vi "WS1050 36 DUT Reliability HD_Cycling Ver1.4.vi"() -> ()   [LabVIEW 2012]
uses:
  WS_VCAP Driver 029/Source/WSVCAP Shell/Type Defs/WSVCAP SHL I2C DUT Mask Mode Enum.ctl
  <vilib>/Utility/file.llb/Read From Spreadsheet File (DBL).vi
  All Driver/Keithley/2012_Keithley 24XX/Keithley 24XX.lvlib
panel:
  out "VISA resource name out":refnum<visa-resource-name>="GPIB0::3::INSTR"
  out "error out 2":errorcluster={"status"=TRUE, "code"=-63192, "source"="niLvFpga_Open_PXI-7813R.vi"}
  in  "Reg1_Bit Cntrl":string[](array[string])=["01", "02", "04", "08", "10", "20", "40", "80", "03", "06", "0C", "D8", "33", "66", "CC", "07", "0E", "1C", "38", "70", "E0", "0F", "1E", "3C", "78", "F0", "1F", "3E", "7C", "F8", "3F", "7E", "FC", "7F", "FE", "FD", "FB", "F7", "EF", "DF", "BF", "7F", "FC", "F9", "F3", "E7", "CF", "9F", "3F", "F8", "F1", "E3", "C7", "8F", "1F", "F0", "E1", "C3", "87", "0F", "E0", "C1", "83", "07", "C0", "81", "03", "AA", "55", "00"]
  out "date string":string="5/19/2014"
  out "PS1 Out":refnum<visa-resource-name>
  out "Ke2000 Out":refnum<visa-resource-name>="GPIB0::9::INSTR"
  in  "VPI_Cmd":string[](array[string])=["000000", "3B3B3B", "000000"]
  in  "VPI Name":string[](array[string])=["All_Drivers OFF", "All Drivers ON", "All Drivers OFF2"]
  in  "Tab Control":T1(tab)
  in  "No of Cmd":i64=3
  in  "Board#":string="BRD5"
  in  "Serial Number":string[][](table)=[["DUT", "SN"], ["DUT1", "1"], ["DUT2", "2"], ["DUT3", "3"], ["DUT4", "4"], ["DUT5", "5"], ["DUT6", "6"], ["DUT7", "7"], ["DUT8", "8"], ["DUT9", "9"], ["DUT10", "10"], ["DUT11", "11"], ["DUT12", "12"], ["DUT13", "13"], ["DUT14", "14"], ["DUT15", "15"], ["DUT16", "16"], ["DUT17", "17"], ["DUT18", "18"], ["DUT19", "19"], ["DUT20", "20"], ["DUT21", "21"], ["DUT22", "22"], ["DUT23", "23"], ["DUT24", "24"], ["DUT25", "25"], ["DUT26", "26"], ["DUT27", "27"], ["DUT28", "28"], ["DUT29", "29"], ["DUT30", "30"], ["DUT31", "31"], ["DUT32", "32"], ["DUT33", "33"], ["DUT34", "34"], ["DUT35", "35"], ["DUT36", "36"]]
  in  "SPI Clock Rate (Hz)":dbl=5000000.0 caption="Cycle Speed" format="%.1p Hz"
  in  "Wafer#":string="T7-EB"
  in  "File Name":string="CYC_WS1050_T7_EB_65C_40V_25DC_EMPTY_BRD5_141017_1"
  in  "TMN DC\\CAP Data Log File Path":path=path "C:/WS1050 36 DUT Data"
  in  "Test Program":string="WS1050 36 DUT Reliability HD_Cycling Ver1.4"
  out "Current Date":string="8/28/2014"
  out "Current Time":string="0950"
  in  "Start Date":string="10/21/2014"
  in  "Start Time":string="1542"
  in  "Comment":string="CYC65C40V"
  in  "OK Button":bool
  in  "Calibration":bool
  in  "Verify CP":bool
  in  "CP Setting":i32(ring) items=["CP OFF", "CP ON", "CP 35V", "CP 40V", "DVA ON", "DVA OFF", "REG1 ON", "REG1 OFF", "REG2 ON", "REG2 OFF", "REG3 ON", "REG3 OFF"]
  in  "Stop Calibration":bool
  in  "Set VDD":dbl=3.3 format="%.3g"
  in  "Command":string[](array[string])=["07020100003B", "070201003B00", "0702013B0000"]
  in  "Clock Rate (Hz)":dbl=1000000.0 caption="Meas Speed" format="%.1p Hz"
  out "AR  Measurent(Hz)":dbl
  in  "PS1 Source":refnum<visa-resource-name>="GPIB0::5::INSTR"
  in  "Ke2000":refnum<visa-resource-name>="GPIB0::9::INSTR"
  in  "CP to HD/Cycle":i32(ring)=1 items=["CP HDC 35V", "CP HDC 40.25V", "CP HDC 27.5V", "CP HDC 30.5V", "CP HDC 44V"]
  out "Simulate FPGA":bool
  out "Online":bool
  out "AR Cycling(Hz)":dbl=5000000.0
  in  "Ke2400":refnum<visa-resource-name>="GPIB0::3::INSTR"
  in  "Initialize AD7747":bool
  in  "DUT Mask Mode":T2=enum."All"
  in  "RFFE Slave Address":u8=7 caption="Slave Address" format="0x%02x"
  out "Activity Log":string="05/19/2014 -- 12:24:35.853::WSVCAP::APP::Application Started\n05/19/2014 -- 12:24:37.606::WSVCAP::WSVCAP SHL::WR I2C-REG:0x0A;MASK:0xFFFFFFFFFFFF;C1 DATA:22:22:22:22:22:22:22:22:22:22:22:22:22:22:22:22;C2 DATA:22:22:22:22:22:22:22:22:22:22:22:22:22:22:22:22;C3 DATA:22:22:22:22:22:22:22:22:22:22:22:22:22:22:22:22\r\n05/19/2014 -- 12:24:37.773::WSVCAP::WSVCAP SHL::WR I2C-ST:0,0,4,1\r\n05/19/2014 -- 12:24:37.903::WSVCAP::WSVCAP SHL::RD I2C-BYTES:4;ADD:0x00;MASK:0xFFFFFFFFFFFF\r\n05/19/2014 -- 12:24:38.045::WSVCAP::WSVCAP SHL::RD I2C:C1 DATA:2:2:2:2:2:2:2:2:2:2:2:2:2:2:2:2|A7:A9:AA:82:82:7F:82:81:82:81:83:82:81:82:82:81|46:36:BB:88:44:A3:E9:2B:32:20:ED:25:BB:3D:68:B|2C:6A:EB:A7:22:56:FE:CC:36:82:D7:B0:3B:48:F9:CC;C2 DATA:2:2:2:2:2:2:2:2:2:2:2:2:2:2:2:2|94:94:94:80:80:80:80:80:81:7E:7E:81:80:7E:80:80|47:33:15:82:62:B:E8:1C:D7:C3:7D:41:7C:B7:4C:2A|C4:B4:AE:8:1E:D1:4E:37:11:C0:6F:63:42:9D:63:B5;C3 DATA:2:2:2:2:2:2:2:2:2:2:2:2:2:2:2:2|95:95:95:81:81:7E:81:80:84:7D:80:83:81:7E:7F:80|AB:C4:14:B5:7B:52:DF:C9:79:5D:5F:30:99:31:1E:F4|6E:5C:F7:A8:C3:EB:7B:EF:33:92:89:77:4D:67:75:DD;STATUS:0:0:4:0\r\n05/19/2014 -- 12:24:38.046::WSVCAP::WSVCAP SHL::WR I2C-REG:0x0A;MASK:0xFFFFFFFFFFFF;C1 DATA:22:22:22:22:22:22:22:22:22:22:22:22:22:22:22:22;C2 DATA:22:22:22:22:22:22:22:22:22:22:22:22:22:22:22:22;C3 DATA:22:22:22:22:22:22:22:22:22:22:22:22:22:22:22:22\r\n05/19/2014 -- 12:24:38.089::WSVCAP::WSVCAP SHL::WR I2C-ST:0,0,4,1\r\n05/19/2014 -- 12:24:38.219::WSVCAP::WSVCAP SHL::RD I2C-BYTES:4;ADD:0x00;MASK:0xFFFFFFFFFFFF\r\n05/19/2014 -- 12:24:38.362::WSVCAP::WSVCAP SHL::RD I2C:C1 DATA:2:2:2:2:2:2:2:2:2:2:2:2:2:2:2:2|A7:AB:AA:82:82:82:83:83:82:82:82:82:7F:82:82:81|4B:32:96:83:3E:61:43:17:25:62:AB:4D:A2:40:2E:5|3C:76:2B:B4:EE:E4:A9:1A:AA:A:26:C7:21:2E:87:5B;C2 DATA:2:2:2:2:2:2:2:2:2:2:2:2:2:2:2:2|94:94:94:80:80:80:80:80:80:7F:80:81:80:80:7F:80|4A:32:19:7D:19:6C:79:46:61:7F:4B:B8:A5:30:F3:14|B4:70:A:8C:9C:DC:43:FA:1E:A:C6:21:A:A9:13:F3;C3 DATA:2:2:2:2:2:2:2:2:2:2:2:2:2:2:2:2|95:97:94:81:80:81:82:81:80:7E:81:84:7F:81:80:80|B2:32:D0:A7:9E:4C:AB:D4:EE:D9:F0:82:B7:91:7:FF|C1:91:B6:3D:D8:E:1B:4F:9F:6A:F1:6C:E7:3F:7:BA;STATUS:0:0:4:0\r\n05/19/2014 -- 12:24:38.364::WSVCAP::WSVCAP SHL::WR I2C-REG:0x0A;MASK:0xFFFFFFFFFFFF;C1 DATA:22:22:22:22:22:22:22:22:22:22:22:22:22:22:22:22;C2 DATA:22:22:22:22:22:22:22:22:22:22:22:22:22:22:22:22;C3 DATA:22:22:22:22:22:22:22:22:22:22:22:22:22:22:22:22\r\n05/19/2014 -- 12:24:38.406::WSVCAP::WSVCAP SHL::WR I2C-ST:0,0,4,1\r\n05/19/2014 -- 12:24:38.536::WSVCAP::WSVCAP SHL::RD I2C-BYTES:4;ADD:0x00;MASK:0xFFFFFFFFFFFF\r\n05/19/2014 -- 12:24:38.678::WSVCAP::WSVCAP SHL::RD I2C:C1 DATA:2:2:2:2:2:2:2:2:2:2:2:2:2:2:2:2|A7:A9:AB:82:82:81:82:82:82:82:82:82:82:82:82:81|46:71:4C:87:43:3D:7F:FC:25:4F:8E:54:97:3E:60:8C|AA:F4:1F:B5:CE:43:1F:36:9:87:9C:78:86:5:B6:8E;C2 DATA:2:2:2:2:2:2:2:2:2:2:2:2:2:2:2:2|94:94:94:80:7F:7F:80:80:80:80:80:81:80:80:80:80|49:36:18:7D:6E:C5:E4:3C:81:2E:41:D3:75:71:E3:72|E8:D3:E6:D1:E0:48:AE:D4:54:D:E8:8E:B4:41:68:4;C3 DATA:2:2:2:2:2:2:2:2:2:2:2:2:2:2:2:2|95:95:95:81:7F:7F:81:81:81:81:81:84:81:81:82:81|B3:F5:90:AB:82:69:7B:93:D0:77:E8:D5:E8:8C:84:E8|B9:AC:EE:2B:B6:71:8F:4A:74:31:56:BB:8A:B7:A0:C8;STATUS:0:0:4:0\r\n05/19/2014 -- 12:24:38.681::WSVCAP::WSVCAP SHL::WR I2C-REG:0x0A;MASK:0xFFFFFFFFFFFF;C1 DATA:22:22:22:22:22:22:22:22:22:22:22:22:22:22:22:22;C2 DATA:22:22:22:22:22:22:22:22:22:22:22:22:22:22:22:22;C3 DATA:22:22:22:22:22:22:22:22:22:22:22:22:22:22:22:22\r\n05/19/2014 -- 12:24:38.723::WSVCAP::WSVCAP SHL::WR I2C-ST:0,0,4,1\r\n05/19/2014 -- 12:24:38.854::WSVCAP::WSVCAP SHL::RD I2C-BYTES:4;ADD:0x00;MASK:0xFFFFFFFFFFFF\r\n05/19/2014 -- 12:24:38.996::WSVCAP::WSVCAP SHL::RD I2C:C1 DATA:2:2:2:2:2:2:2:2:2:2:2:2:2:2:2:2|A7:A9:AA:82:82:7F:83:81:82:81:84:82:7F:82:7F:82|43:FB:E:7F:3C:AD:35:35:26:A2:6C:21:4B:3D:8:6|63:9A:E1:F3:95:32:91:42:90:3C:78:1F:5C:D7:5F:D8;C2 DATA:2:2:2:2:2:2:2:2:2:2:2:2:2:2:2:2|94:94:94:80:80:80:80:80:81:80:7E:81:80:7E:7F:80|48:36:18:7F:5E:3D:69:83:DE:AE:A1:9E:31:AE:BB:96|15:A0:44:17:13:FD:CC:C8:6D:B2:EF:A7:C:C7:3B:F;C3 DATA:2:2:2:2:2:2:2:2:2:2:2:2:2:2:2:2|95:96:94:81:81:7E:82:80:84:80:80:84:7F:7E:7D:82|AD:3B:6D:A9:7C:57:9D:F5:7A:96:23:5C:36:2D:ED:5A|CD:46:DB:3B:C7:BD:70:60:33:B8:B:F7:63:A:51:4D;STATUS:0:0:4:0\r\n05/19/2014 -- 12:24:38.998::WSVCAP::WSVCAP SHL::WR I2C-REG:0x0A;MASK:0xFFFFFFFFFFFF;C1 DATA:22:22:22:22:22:22:22:22:22:22:22:22:22:22:22:22;C2 DATA:22:22:22:22:22:22:22:22:22:22:22:22:22:22:22:22;C3 DATA:22:22:22:22:22:22:22:22:22:22:22:22:22:22:22:22\r\n05/19/2014 -- 12:24:39.040::WSVCAP::WSVCAP SHL::WR I2C-ST:0,0,4,1\r\n05/19/2014 -- 12:24:39.170::WSVCAP::WSVCAP SHL::RD I2C-BYTES:4;ADD:0x00;MASK:0xFFFFFFFFFFFF\r\n05/19/2014 -- 12:24:39.311::WSVCAP::WSVCAP SHL::RD I2C:C1 DATA:2:2:2:2:2:2:2:2:2:2:2:2:2:2:2:2|A7:AA:AB:82:82:81:82:81:82:81:82:82:82:82:7F:82|44:F1:90:87:45:44:C8:2C:2C:F1:FC:1B:94:3B:3C:75|4A:49:95:19:99:73:64:3:23:24:F3:A2:5E:7F:C4:B6;C2 DATA:2:2:2:2:2:2:2:2:2:2:2:2:2:2:2:2|94:94:94:80:80:80:80:7F:80:80:7E:80:80:7E:7F:80|4C:36:17:7D:A8:9F:DE:C7:53:6D:8A:F4:41:A5:C6:E0|90:2E:24:C:D9:22:E4:76:3B:40:1D:53:33:B1:3E:4D;C3 DATA:2:2:2:2:2:2:2:2:2:2:2:2:2:2:2:2|95:97:95:81:81:7F:81:80:80:81:7F:82:81:7E:7D:82|AE:2B:A7:AB:CC:CD:A4:38:FD:17:80:F2:92:2D:45:C4|76:E5:D:B9:AD:B5:BA:8D:28:32:9E:42:B7:20:4A:D9;STATUS:0:0:4:0\r\n05/19/2014 -- 12:24:39.313::WSVCAP::WSVCAP SHL::WR I2C-REG:0x0A;MASK:0xFFFFFFFFFFFF;C1 DATA:22:22:22:22:22:22:22:22:22:22:22:22:22:22:22:22;C2 DATA:22:22:22:22:22:22:22:22:22:22:22:22:22:22:22:22;C3 DATA:22:22:22:22:22:22:22:22:22:22:22:22:22:22:22:22\r\n05/19/2014 -- 12:24:39.355::WSVCAP::WSVCAP SHL::WR I2C-ST:0,0,4,1\r\n05/19/2014 -- 12:24:39.486::WSVCAP::WSVCAP SHL::RD I2C-BYTES:4;ADD:0x00;MASK:0xFFFFFFFFFFFF\r\n05/19/2014 -- 12:24:39.628::WSVCAP::WSVCAP SHL::RD I2C:C1 DATA:2:2:2:2:2:2:2:2:2:2:2:2:2:2:2:2|A7:A9:AA:82:82:82:83:82:82:82:82:82:7F:82:7F:82|47:18:E4:87:3E:E7:6:65:25:92:37:38:A8:3E:89:85|7C:A7:7:2B:A3:7A:EC:EF:89:ED:F4:D3:D8:BC:3A:F5;C2 DATA:2:2:2:2:2:2:2:2:2:2:2:2:2:2:2:2|94:94:94:80:7F:80:80:7F:81:80:7E:80:80:80:81:80|49:37:17:80:76:25:6A:F8:DF:55:97:4D:B8:5B:2B:B1|13:E3:9A:3E:1A:2D:4F:B6:DB:E9:61:FA:8B:D6:9:CC;C3 DATA:2:2:2:2:2:2:2:2:2:2:2:2:2:2:2:2|95:95:95:81:7F:80:82:81:84:80:7F:81:80:81:7F:82|AF:93:3B:AF:5B:11:82:E4:7E:C3:2D:72:9:96:D9:A|DB:96:F2:10:5F:64:9A:C6:98:12:27:7D:10:D3:20:D9;STATUS:0:0:4:0\r\n05/19/2014 -- 12:24:40.132::WSVCAP::WSVCAP SHL::CLOSE\r\n"
  in  "C1 Cap DAC":u8=128 caption="B Data In" format="0x%02x"
  in  "C2 Cap DAC":u8=128 caption="B Data In" format="0x%02x"
  in  "C3 Cap DAC":u8=128 caption="B Data In" format="0x%02x"
  out "IDD Brd(uA)":string
  in  "CP to Meas":i32(ring)=1 items=["CP HDC 35V", "CP HDC 40.25V", "CP HDC 27.5V", "CP HDC 30.5V", "CP HDC 44V"]
  in  "CP VPI":i32(ring) items=["CP HDC 35V", "CP HDC 40.25V", "CP HDC 27.5V", "CP HDC 30.5V", "CP HDC 44V"]
  in  "Repeat Meas(s)":u32=900
  in  "Real No. From\nLookup Table":bool
  in  "Control Panel":T3={"Verify Socket"=FALSE, "HD/CYC"=FALSE, "E-CAL"=FALSE, "DVA"=FALSE, "VPI"=TRUE, "VSA"=TRUE, "HS"=TRUE}
  out "Verify Socket":bool
  out "HD/CYC":bool
  out "E-CAL":bool
  out "DVA":bool
  out "VPI":bool
  out "VSA":bool
  out "HS":bool
  in  "Lot#":string="WS1050"
  out "AD7747 Values":string[][](table)
  in  "Freq(Hz)":string="12K"
  in  "Reset P/S":bool
  in  "WS1050/51":bool=TRUE
  in  "CP with DVA ON":i32(ring) items=["CP HDC 35V", "CP HDC 40.25V", "CP HDC 27.5V", "CP HDC 30.5V", "CP HDC 44V"]
  in  "% Duty Cycle":string="33"
  in  "Cmd To HD":string="0702013B3B3B"
  in  "Post CMd Delay":dbl[](array[numeric])=[1.8e-05, 1.8e-05, 1.8e-05] min=0.0 max=0.5 format="%#.0p s"
  in  "Cmin/Act":bool=TRUE
  in  "Test Seq":i32(ring)=3 items=["C1_C2_C3", "C2_C1_C3", "C3_C2_C1", "ALL"]
  out "40V_1":string[][](table)
  out "NOM IDD OFF(uA)":string
  out "40V_2":string[][](table)
  out "40V_3":string[][](table)
  out "Total Time":u64
  in  "Set HD/Cycle \nto Complete":u64=50000000000
  out "No of HD/Cycle\nCompleted":u64
  out "Cycle Count":u64 min=1 max=4 step=1
  out "Loop \ncompleted":i32=1
  out "Previous Time":string="12:20:26 PM"
  out "STATUS":string="Idle...."
  out "Total Delta C2(pF)":string[](array[string])
  out "Total Delta C1(pF)":string[](array[string])
  out "Total Delta C3(pF)":string[](array[string])
  out "RB Reg for HD":string[](array[string])
  out "RB Reg for HD/Cycle":string[](array[string])
  out "VPI C2":string[][](table)
  out "VPI C3":string[][](table)
  out "NOM IDD ON (uA)":string
  out "IDD_HD/CYC (uA)":string="164.601255E+0"
  in  "stop During HD/Cycles":bool
  in  "stop":bool
  out "IDD Stdby(uA)":string="2.606990E+0"
  out "VPI C1":string[][](table)
  out "VSA_V1":string[][](table)
  out "VSA_V2":string[][](table)
  out "VSA_V3":string[][](table)
  in  "VSA Voltage(V)":dbl[](array[numeric])=[-10.0, 0.0, 10.0]
  in  "DC_Temp":i32=65
  in  "HD/CYC Temp":i32=65
  in  "Time All ON (s)":u32=120
  in  "Time All OFF (s)":u32=120
  in  "HD_DC (Min)":u64=259200
  out "LPs Count":i32
  in  "X Repeat":i32=100
  out "No LPs to RP":i32
  out "Run Loops":i32=1
  out "TTCompleted":u64=2000
  in  "TTF Completed":u64=50000000000
  out "% Delta C_T0":string[][](array[string])
  out "% Delta C":string[][](array[string])
  out "EFuse RB T0":string[](array[string])
  out "Current EFuse Read back":string[](array[string])
  out "EFuse Readback Status":bool[](array[boolean])
  in  "DeltaC Target Setting(pF)":dbl=7.375
  out "error out":errorcluster
  in  "error in (no error)":errorcluster
  in  "HD RP":dbl=60.0
  in  "Cycle RP":dbl=10000.0
  out "Min Plot_1":dbl[][](graph) caption="(Y) Multi Plot 2"
  out "Min Plot_2":dbl[][](graph) caption="(Y) Multi Plot 2"
  out "Min Plot_3":dbl[][](graph) caption="(Y) Multi Plot 2"
  in  "Debug":bool
  in  "No of Rows\nFrom Spread Sheet":i32
  in  "Plot Delta Cmin":bool=TRUE
  in  "Plot":T4(ring)
  # "Company:  WiSpry Inc\n20 Fairbanks Ste 198 Irvine CA 92618\n\nAuthor:  Andy V Tran\nCreated:  04/21/2015\nLabVIEW 2012 Pro\nTest Program:  WS1050 36 DUT Reliability HD_Cycling ver1.4\nFPGA: WS_VCAP Driver 029"
  # "Note for HD Duty Cycle:\n1.  Set time to start HD_DC (Min), default is 259200 (6 months) \n2.  Set Time for Duty Cycle ON/OFF, default setting is 2 minutes\n3.  No of Loops to RP = 3600s/(Time ALL ON(s) + Time ALL + OFF(s))\n4.  Set X Repeat = no of runs, default is 100 runs\n5.  Set TTF Completed to stop the test.\n\nVer 1.4\n1.  Make measurement of C1, C2 and C3 at the same time"
  # "Minutes"
  # "X1000"
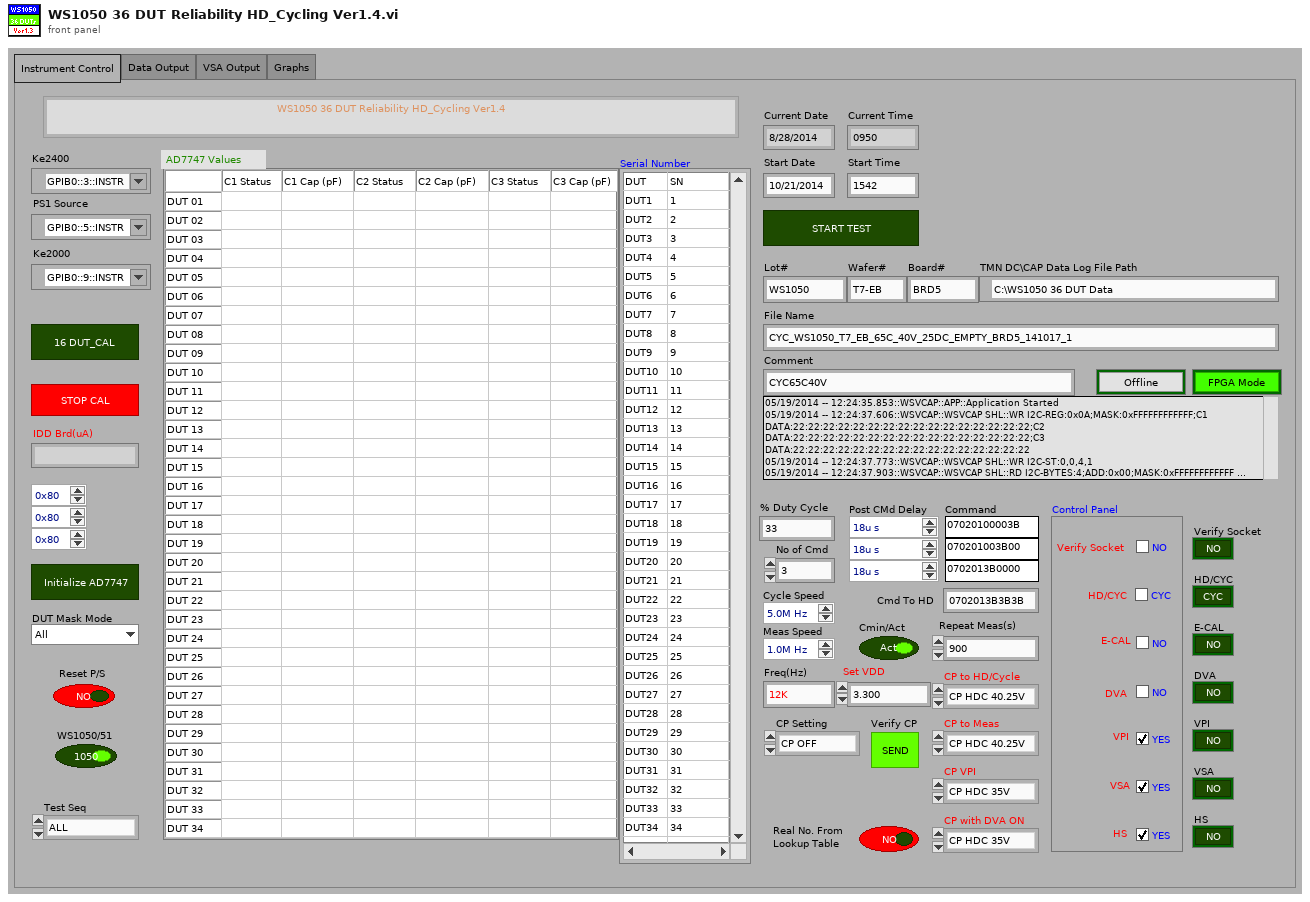
[diagram p1: front panel]
types:
  T1 = enum32{"Instrument Control", "Data Output", "VSA Output", "Graphs"}
  T2 = typedef "WSVCAP SHL I2C DUT Mask Mode Enum.ctl" = enum16{"Custom", "C1", "C2", "C3", "All"}
  T3 = cluster{"Verify Socket":bool, "HD/CYC":bool, "E-CAL":bool, "DVA":bool, "VPI":bool, "VSA":bool, "HS":bool}
  T4 = enum16{"ALL DUTs", "DUT 01", "DUT 02", "DUT 03", "DUT 04", "DUT 05", "DUT 06", "DUT 07", "DUT 08", "DUT 09", "DUT 10", "DUT 11", "DUT 12", "DUT 13", "DUT 14", "DUT 15", "DUT 16", "DUT 17", "DUT 18", "DUT 19", "DUT 20", "DUT 21", "DUT 22", "DUT 23", "DUT 24", "DUT 25", "DUT 26", "DUT 27", "DUT 28", "DUT 29", "DUT 30", "DUT 31", "DUT 32", "DUT 33", "DUT 34", "DUT 35", "DUT 36"}
  T5 = typedef "WSVCAP SHL Core System Cluster.ctl" = cluster{"Settings":T6, "FPGA Resource":tag, "Online":bool, "I2C Wait Ticks":u32, "SPI Wait Ticks":u32, "RFFE Wait Ticks":u32}
  T6 = typedef "WSVCAP SHL I2C Settings Cluster.ctl" = cluster{"FPGA Resource Name":string, "I2C Slave Address":u8, "I2C Clock Rate (Hz)":dbl, "SPI Clock Rate (Hz)":dbl, "RFFE Slave Address":u8, "RFFE Clock Rate (Hz)":dbl, "Simulate FPGA":bool, "C1 Cap DAC Default":u8, "C2 Cap DAC Default":u8, "C3 Cap DAC Default":u8}
  T7 = enum16{"Idle...", "Voltage 1", "Voltage 2", "Voltage 3"}[]
  T8 = cluster{"Test Program ":string, "Comment":string, "Data Out":string, "Data Out":string, "Data Out":string, string, "Data Out":string, "Data Out":string, "string":string, "Freq(Hz)":string, "Board#":string}
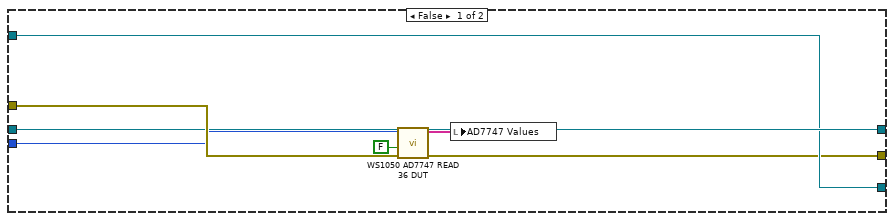
[diagram p10: hidden frame]
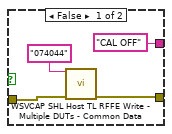
[diagram p11: hidden frame]
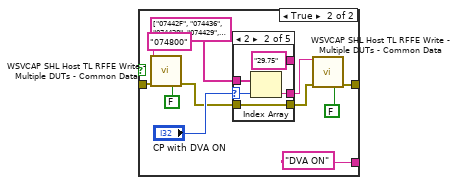
[diagram p12: hidden frame]
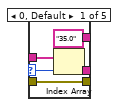
[diagram p13: hidden frame]
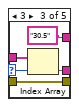
[diagram p14: hidden frame]
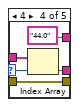
[diagram p15: hidden frame]
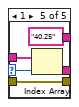
[diagram p16: hidden frame]
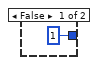
[diagram p17: hidden frame]
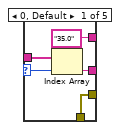
[diagram p18: hidden frame]
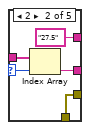
[diagram p19: hidden frame]
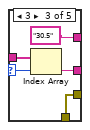
[diagram p20: hidden frame]
diagram:
  w19 = TRUE
  w25 = u16 0 items=["Off", "Moving Filter", "Repeating Filter"] ("Digital Filter (0: Off)")
  w26 = u16 7 items=["3.5 Digits"=4, "4.5 Digits"=5, "5.5 Digits"=6, "6.5 Digits"=7] ("Resolution (7: 6.5 digits)")
  n1 = case shown="True" w19 {
    tunnel: "error in (no error)" -> [w33 w34]
    tunnel: [w33 w41] -> w5
    frame False {
    }
    frame True {
      n2 = call "WSVCAP SHL Host TL Initialize.vi"("error in"=w34) -> ("error out"=w35:errorcluster)  [unwired: 13 in, 1 out]
      n3 = control-ref of="Activity Log"() -> (w37:refnum<vi>)
      n4 = call "ACT LG Activity Log Core.vi"("Display Ref"=w37, "Source"="WSVCAP", "Error In (no error)"=w35) -> ("Error Out"=w36:errorcluster)  [unwired: 11 in, 1 out]
      n5 = call "WSVCAP SHL Host TL Status Manager.vi"("error in"=w36) -> ("System Out"=w42:T5, "error out"=w41:errorcluster)  [unwired: 13 in]
      n6 = Unbundle By Name(w42) -> ("Online"=→"Online":bool, "Settings.Simulate FPGA"=→"Simulate FPGA":bool)
    }
  }
  n7 = case shown="True" TRUE {
    tunnel: w5 -> [w43 w48]
    tunnel: [w44 w47] -> w16
    tunnel: [w43 w46] -> w9
    tunnel: "Ke2400" -> [w44 w45]
    frame False {
    }
    frame True {
      n8 = VISA Write(VISA resource name=w45, write buffer="SOUR:FUNC VOLT;VOLT:MODE FIX;RANG 100;LEV 0.0;:SENS:FUNC \"CURR\";CURR:PROT 60E-3;RANG 100E-3;:OUTP ON", error in (no error)=w48) -> (VISA resource name out=w47:refnum<visa-resource-name>, error out=w46:errorcluster)  [unwired: 1 out]
    }
  }
  n9 = case shown="True" "Reset P/S" {
    tunnel: "PS1 Source" -> [w50 w57]
    tunnel: [w50 w55] -> w30
    tunnel: w5 -> [w51 w53]
    tunnel: [w51 w52] -> w4
    frame False {
    }
    frame True {
      n10 = call "Agilent 3631A Initialize.vi"("error in (no error)"=w53, "Default"=FALSE ("Reset? (T: Yes)"), "Reset"=TRUE ("ID Query? (T: Yes)"), "VISA resource name"=w57) -> ("error out"=w52:errorcluster, "VISA resource name out"=w55:refnum<visa-resource-name>)  [unwired: 6 in]
    }
  }
  n11 = call "Ke2000 Initialize.vi"("error in (no error)"=w5, "VISA resource name"="Ke2000") -> ("error out"=w27:errorcluster, "VISA resource name out"=w28:refnum<visa-resource-name>)  [unwired: 8 in]
  n12 = call "Ke2000 Configure DC Current.vi"("Resolution (7: 6.5 digits)"=w26, "Digital Filter (0: Off)"=w25, "Auto Range? (T: Auto)"=FALSE, "error in (no error)"=w27, "Custom Range (0 A)"=1.0, "VISA resource name"=w28) -> ("error out"=w6:errorcluster, "VISA resource name out"=w23:refnum<visa-resource-name>)  [unwired: 4 in]
  n13 = case shown="True" TRUE {
    tunnel: [_ w58] -> w32
    frame False {
    }
    frame True {
      n14 = call-poly <vilib>:"Read From Spreadsheet File.vi"("number of rows (all:-1)"=-1) -> ("all rows"=w58:dbl[][])  [unwired: 6 in, 4 out]
    }
  }
  n15 = Merge Errors(w9, w6, w4) -> (w17:errorcluster)
  n16 = while {
    tunnel: w17 -> [w62]
    tunnel: [w71] -> w13
    tunnel: w32 -> [w87]
    tunnel: w30 -> [w75]
    tunnel: w23 -> [w76]
    tunnel: [w85] -> w22
    tunnel: [w84] -> w21
    tunnel: w16 -> [w82]
    tunnel: [w81] -> w14
    tunnel: [FALSE ("stop")] -> w7
    i -> [w83]
    stop <- w88 stop-if-true
    n17 = case shown="0" w83 {
      tunnel: w62 -> [w99 w101]
      tunnel: [w98 w101] -> w78
      tunnel: "RFFE Slave Address" -> [w96 _]
      frame 0 {
        w92 = dbl[][] []
        w91 = "" ("uA")
        w93 = string[][] []
        w94 = string[] [] ("EFuse Read back")
        w100 = u64 0 ("No of HD/Cycle\nCompleted")
        n18 = local write "RB Reg for HD/Cycle"(w94) -> ()
        n19 = local write "Current EFuse Read back"(w94) -> ()
        n20 = local write "EFuse RB T0"(w94) -> ()
        n21 = local write "Total Delta C1(pF)"(w94) -> ()
        n22 = local write "Total Delta C2(pF)"(w94) -> ()
        n23 = local write "Total Delta C3(pF)"(w94) -> ()
        n24 = local write "No of HD/Cycle\nCompleted"(w100) -> ()
        n25 = local write "Cycle Count"(w100) -> ()
        n26 = local write "VPI C2"(w93) -> ()
        n27 = local write "VSA_V3"(w93) -> ()
        n28 = local write "VSA_V1"(w93) -> ()
        n29 = local write "40V_2"(w93) -> ()
        n30 = local write "40V_1"(w93) -> ()
        n31 = local write "NOM IDD OFF(uA)"(w91) -> ()
        n32 = local write "NOM IDD ON (uA)"(w91) -> ()
        n33 = local write "IDD Brd(uA)"(w91) -> ()
        n34 = local write "VSA_V2"(w93) -> ()
        n35 = local write "VPI C1"(w93) -> ()
        n36 = local write "VPI C3"(w93) -> ()
        n37 = local write "% Delta C"(w93) -> ()
        n38 = local write "% Delta C_T0"(w93) -> ()
        n39 = local write "40V_3"(w93) -> ()
        n40 = call "WSVCAP SHL Host TL RFFE Configure.vi"("RFFE Slave Address"=w96, "Clock Rate (Hz)"="Clock Rate (Hz)", "error in"=w99) -> ("Actual Rate (Hz)"=→"AR  Measurent(Hz)":dbl, "error out"=w98:errorcluster)  [unwired: 11 in]
        n41 = local write "Min Plot_3"(w92) -> ()
        n42 = local write "Min Plot_1"(w92) -> ()
        n43 = local write "Min Plot_2"(w92) -> ()
      }
      frame 1, Default {
      }
    }
    n44 = while {
      tunnel: ["stop"] -> w80
      tunnel: w78 -> [w127]
      tunnel: [w119] -> w72
      tunnel: w75 -> [w126]
      tunnel: w76 -> [w121]
      tunnel: [w122] -> w74
      tunnel: [w120] -> w73
      tunnel: [w117] -> w69
      tunnel: [w116] -> w68
      tunnel: [w115] -> w67
      tunnel: [w114] -> w66
      tunnel: [w113] -> w65
      tunnel: [w112] -> w64
      tunnel: [w111] -> w63
      tunnel: ["Command"] -> w61
      tunnel: ["Post CMd Delay"] -> w60
      stop <- w134 stop-if-true
      # "Set Date & Time to Start Test"
      n45 = case shown="True" "Initialize AD7747" {
        tunnel: w127 -> [w143 w148]
        tunnel: [w143 w144] -> w110
        tunnel: w126 -> [w142 w146]
        tunnel: [w142 w145] -> w125
        frame False {
        }
        frame True {
          w149 = T7 [enum."Voltage 2", enum."Voltage 3", enum."Voltage 1"] items=["Idle...", "Voltage 1", "Voltage 2", "Voltage 3"]
          n46 = for {
            tunnel: w146 -> [w159]
            tunnel: w149 -> [w157] mode=indexing
            tunnel: [w156] -> w145
            shift-right: [w152] -> w147
            shift-left: w148 -> [w160]
            n47 = local read "Set VDD"() -> (w155:dbl)
            n48 = call "E3631A_Voltage Controller.vi"("VISA resource name"=w159, "I_VDD(A)"=0.5, "Channel Controller"=w157, "Voltage 1"=w155, "Voltage 2"=3.3, "error in (no error)"=w160, "I_3.3V (A)"=0.5) -> ("VISA resource name out"=w156:refnum<visa-resource-name>, "error out"=w151:errorcluster)  [unwired: 7 in]
            n49 = call "Delay T4.vi"("milliseconds to wait"=u32 100, "error in (no error)"=w151) -> ("error out"=w152:errorcluster)  [unwired: 9 in]
          }
          n50 = call "WS1050_AD7747_Init 36DUT.vi"("error in"=w147) -> ("error out"=w144:errorcluster)  [unwired: 10 in]
        }
      }
      n51 = call "Time_stamp.vi"() -> ("date/time string"=w139:string, "date string"=w141:string)  [unwired: 2 in]
      "Current Date" <- w141
      "Current Time" <- w139
      n52 = Equal?(x=w141, y="Start Date") -> (x = y?=w137:bool)
      n53 = Equal?(x=w139, y="Start Time") -> (x = y?=w136:bool)
      n54 = And(x=w137, y=w136) -> (x .and. y?=w133:bool)
      n55 = Compound Arithmetic op=OR(w133, "OK Button", "stop") -> (w134:bool)
      n56 = case shown="True" "Calibration" {
        tunnel: w110 -> [w190 w207]
        tunnel: [w184 w204] -> w108
        tunnel: w125 -> [w189 w203]
        tunnel: "DUT Mask Mode" -> [w188 w199]
        tunnel: [w189 w198] -> w123
        tunnel: w121 -> [w187 w194]
        tunnel: [w187 w191] -> w120
        frame False {
          n57 = call "WS1050 AD7747 READ 36 DUT.vi"("error in"=w190, "Log (T)"=FALSE, "DUT Mask Mode (All)"=w188) -> ("error out"=w184:errorcluster, "AD7747 Values"=w185:string[][])  [unwired: 7 in]
          n58 = local write "AD7747 Values"(w185) -> ()
        }
        frame True {
          n59 = flat-sequence {
            tunnel: w207 -> [w216]
            tunnel: [w211] -> w206
            tunnel: w203 -> [w215]
            tunnel: [w214] -> w202
            tunnel: w199 -> [w213]
            tunnel: [w213] -> w200
            tunnel: w194 -> [w209]
            tunnel: [w208] -> w193
            tunnel: w206 -> [w240]
            tunnel: [w239] -> w205
            tunnel: w202 -> [w238]
            tunnel: [w238] -> w201
            tunnel: w200 -> [w237]
            tunnel: "C1 Cap DAC" -> [w233]
            tunnel: "C2 Cap DAC" -> [w232]
            tunnel: "C3 Cap DAC" -> [w231]
            tunnel: w193 -> [w230]
            tunnel: [w230] -> w192
            tunnel: w205 -> [w249]
            tunnel: [w252] -> w204
            tunnel: w201 -> [w251]
            tunnel: [w248] -> w198
            tunnel: w192 -> [w247]
            tunnel: [w247] -> w191
            frame #0 {
              w217 = T7 [enum."Voltage 2", enum."Voltage 3", enum."Voltage 1"] items=["Idle...", "Voltage 1", "Voltage 2", "Voltage 3"]
              n60 = for {
                tunnel: w215 -> [w228]
                tunnel: w217 -> [w226] mode=indexing
                tunnel: [w225] -> w214
                shift-right: [w223] -> w210
                shift-left: w216 -> [w229]
                n61 = local read "Set VDD"() -> (w220:dbl)
                n62 = call "E3631A_Voltage Controller.vi"("VISA resource name"=w228, "I_VDD(A)"=0.5, "Channel Controller"=w226, "Voltage 1"=w220, "Voltage 2"=3.3, "error in (no error)"=w229, "I_3.3V (A)"=0.5) -> ("VISA resource name out"=w225:refnum<visa-resource-name>, "error out"=w222:errorcluster)  [unwired: 7 in]
                n63 = call "Delay T4.vi"("milliseconds to wait"=u32 100, "error in (no error)"=w222) -> ("error out"=w223:errorcluster)  [unwired: 9 in]
              }
              n64 = call "Ke2000 Single Reading.vi"("error in (no error)"=w210, "VISA resource name"=w209) -> ("error out"=w211:errorcluster, "VISA resource name out"=w208:refnum<visa-resource-name>, "uA"=→"IDD Brd(uA)":string)  [unwired: 5 in, 2 out]
              n65 = One Button Dialog(message="Please verify all sockets should be empty...") -> ()  [unwired: 1 in, 1 out]
            }
            frame #1 {
              n66 = call "WS1050 CAPDAC Setting.vi"("DUT Mask Mode (All)"=w237, "error in"=w240, "C3 Cap DAC"=w231, "C2 Cap DAC"=w232, "C1 Cap DAC"=w233) -> ("error out"=w235:errorcluster)  [unwired: 5 in, 1 out]
              n67 = call "WS1050 OFFSET CAL.vi"("error in"=w235, "OFFSET CAL"=TRUE ("Read?")) -> ("error out"=w234:errorcluster)  [unwired: 8 in, 1 out]
              n68 = while {
                tunnel: w234 -> [w246]
                tunnel: [w245] -> w239
                tunnel: w237 -> [w243]
                stop <- "Stop Calibration" stop-if-true
                n69 = call "WS1050 AD7747 READ 36 DUT.vi"("error in"=w246, "Log (T)"=FALSE, "DUT Mask Mode (All)"=w243) -> ("error out"=w245:errorcluster, "AD7747 Values"=→"AD7747 Values":string[][])  [unwired: 7 in]
              }
            }
            frame #2 {
              w250 = T7 [enum."Voltage 2", enum."Voltage 3", enum."Voltage 1"] items=["Idle...", "Voltage 1", "Voltage 2", "Voltage 3"]
              n70 = for {
                tunnel: w251 -> [w264]
                tunnel: w250 -> [w261] mode=indexing
                tunnel: [w260] -> w248
                shift-right: [w256] -> w252
                shift-left: w249 -> [w262]
                n71 = call "E3631A_Voltage Controller.vi"("VISA resource name"=w264, "I_VDD(A)"=0.5, "Channel Controller"=w261, "Voltage 1"=0.0, "Voltage 2"=3.3, "error in (no error)"=w262, "I_3.3V (A)"=0.5) -> ("VISA resource name out"=w260:refnum<visa-resource-name>, "error out"=w255:errorcluster)  [unwired: 7 in]
                n72 = call "Delay T4.vi"("milliseconds to wait"=u32 100, "error in (no error)"=w255) -> ("error out"=w256:errorcluster)  [unwired: 9 in]
              }
              n73 = One Button Dialog(message="Calibration Completed....") -> ()  [unwired: 1 in, 1 out]
            }
          }
        }
      }
      n74 = call "Control Panel.vi"("error in (no error)"=w110, "Control Panel"="Control Panel") -> ("error out"=w107:errorcluster, "VPI"=w113:bool, "DVA"=w114:bool, "E-CAL"=w115:bool, "VSA"=w112:bool, "HD/CYC"=w116:bool, "HS"=w111:bool, "Verify Socket"=w117:bool)  [unwired: 2 in]
      "Verify Socket" <- w117
      "E-CAL" <- w115
      "VPI" <- w113
      "VSA" <- w112
      "HS" <- w111
      "HD/CYC" <- w116
      "DVA" <- w114
      n75 = Merge Errors(w107, w108) -> (w109:errorcluster)
      n76 = case shown="True" "Verify CP" {
        tunnel: [w161 w165] -> w119
        tunnel: w123 -> [w162 w168]
        tunnel: [w162 w166] -> w122
        tunnel: w109 -> [w161 w164]
        frame False {
        }
        frame True {
          w169 = T7 [enum."Voltage 2", enum."Voltage 3", enum."Voltage 1"] items=["Idle...", "Voltage 1", "Voltage 2", "Voltage 3"]
          # "Verify CP"
          n77 = for {
            tunnel: w168 -> [w182]
            tunnel: w169 -> [w180] mode=indexing
            shift-right: [w177] -> w167
            shift-left: w164 -> [w183]
            tunnel: [w175] -> w166
            n78 = local read "Set VDD"() -> (w179:dbl)
            n79 = call "E3631A_Voltage Controller.vi"("VISA resource name"=w182, "I_VDD(A)"=0.5, "Channel Controller"=w180, "Voltage 1"=w179, "Voltage 2"=3.3, "error in (no error)"=w183, "I_3.3V (A)"=0.5) -> ("VISA resource name out"=w175:refnum<visa-resource-name>, "error out"=w178:errorcluster)  [unwired: 7 in]
            n80 = call "Delay T4.vi"("milliseconds to wait"=u32 100, "error in (no error)"=w178) -> ("error out"=w177:errorcluster)  [unwired: 9 in]
          }
          n81 = Index Array(array=string[] ["074000", "074040", "07476F", "074776", "074800", "074820", "07413B", "074100", "07423B", "074200", "07433B", "074300"], index="CP Setting") -> (element=w170:string)
          n82 = call "WSVCAP SHL Host TL RFFE Write - Multiple DUTs - Common Data.vi"("Data Out"=w170, "error in"=w167, "Log (T)"=FALSE) -> ("error out"=w165:errorcluster)  [unwired: 12 in]
        }
      }
      n83 = Array Subset(array="Post CMd Delay", length="No of Cmd") -> (w105:dbl[])  [unwired: 1 in]
      n84 = Array Subset(array="Command", length="No of Cmd") -> (w106:string[])  [unwired: 1 in]
      n85 = property on="Post CMd Delay" class="Arr (strict)"("Number of Rows"="No of Cmd") -> ()  [unwired: 2 in, 2 out]
      n86 = local write "Command"(w106) -> ()
      n87 = local write "Post CMd Delay"(w105) -> ()
      n88 = property on="Command" class="Arr (strict)"("Number of Rows"="No of Cmd") -> ()  [unwired: 2 in, 2 out]
      n89 = Wait Until Next ms Multiple(millisecond multiple=u32 100) -> ()  [unwired: 1 out]
    }
    n90 = case shown="False" w80 {
      tunnel: w72 -> [w324 w1878]
      tunnel: [w309 w1878] -> w71
      tunnel: w87 -> [w325 _]
      tunnel: w74 -> [w323 w1876]
      tunnel: w73 -> [w315 w1877]
      tunnel: [w321 w1877] -> w85
      tunnel: [w319 w1876] -> w84
      tunnel: w82 -> [w312 w1875]
      tunnel: [w308 w1875] -> w81
      tunnel: "RFFE Slave Address" -> [w303 _]
      tunnel: [FALSE ("stop During HD/Cycles") FALSE ("stop During HD/Cycles")] -> w70
      tunnel: w69 -> [w278 _]
      tunnel: w68 -> [w277 _]
      tunnel: w67 -> [w276 _]
      tunnel: w66 -> [w275 _]
      tunnel: w65 -> [w274 _]
      tunnel: w64 -> [w273 _]
      tunnel: w63 -> [w272 _]
      tunnel: w61 -> [w266 _]
      tunnel: w60 -> [w265 _]
      frame False {
        w304 = u64 0 ("Total Completed")
        w283 = u32 100 ("milliseconds to wait")
        w320 = T7 [enum."Voltage 2", enum."Voltage 3", enum."Voltage 1"] items=["Idle...", "Voltage 1", "Voltage 2", "Voltage 3"]
        w322 = T7 [enum."Voltage 2", enum."Voltage 3", enum."Voltage 1"] items=["Idle...", "Voltage 1", "Voltage 2", "Voltage 3"]
        # "VSA"
        # "HS"
        # "HD/CYC"
        # "DVA"
        # "E-CAL"
        # "VPI"
        # "Verify Socket"
        n91 = for {
          tunnel: w324 -> [w1873]
          tunnel: w323 -> [w1872]
          tunnel: w322 -> [w1870] mode=indexing
          tunnel: [w1865] -> w317
          tunnel: [w1869] -> w307
          n92 = local read "Set VDD"() -> (w1868:dbl)
          n93 = call "E3631A_Voltage Controller.vi"("VISA resource name"=w1872, "I_VDD(A)"=0.5, "Channel Controller"=w1870, "Voltage 1"=w1868, "Voltage 2"=3.3, "error in (no error)"=w1873, "I_3.3V (A)"=0.5) -> ("VISA resource name out"=w1869:refnum<visa-resource-name>, "error out"=w1866:errorcluster)  [unwired: 7 in]
          n94 = call "Delay T4.vi"("milliseconds to wait"=u32 100, "error in (no error)"=w1866) -> ("error out"=w1865:errorcluster)  [unwired: 9 in]
        }
        n95 = local write "Total Time"(w304) -> ()
        n96 = local write "TTCompleted"(w304) -> ()
        n97 = call "WSVCAP SHL Host TL RFFE Write - Multiple DUTs - Common Data.vi"("Data Out"="074000", "error in"=w317, "Log (T)"=FALSE) -> ("error out"=w318:errorcluster)  [unwired: 12 in]
        n98 = local read "IDD Brd(uA)"() -> (w292:string)
        n99 = call "Delay T4.vi"("milliseconds to wait"=w283, "error in (no error)"=w318) -> ("error out"=w316:errorcluster)  [unwired: 9 in]
        n100 = call "Ke2000 Single Reading.vi"("error in (no error)"=w316, "VISA resource name"=w315) -> ("error out"=w293:errorcluster, "VISA resource name out"=w314:refnum<visa-resource-name>, "uA"=w295:string)  [unwired: 5 in, 2 out]
        n101 = call "Substration.vi"("error in (no error)"=w293, "Input2"=w292, "Input1"=w295) -> ("error out"=w268:errorcluster, "In1 - In2"=w294:string)  [unwired: 7 in]
        "IDD Stdby(uA)" <- w294
        n102 = case shown="True" w277 {
          tunnel: [1 ("X Repeat") w386] -> w306
          frame False {
          }
          frame True {
            n103 = local read "X Repeat"() -> (w386:i32)
          }
        }
        n104 = call "WSVCAP SHL Host TL RFFE Write - Multiple DUTs - Common Data.vi"("Data Out"="074040", "error in"=w268, "Log (T)"=FALSE) -> ("error out"=w267:errorcluster)  [unwired: 12 in]
        n105 = call "Delay T4.vi"("milliseconds to wait"=w283, "error in (no error)"=w267) -> ("error out"=w301:errorcluster)  [unwired: 9 in]
        n106 = case shown="False" w275 {
          tunnel: w301 -> [w348 w357]
          tunnel: [w347 w355] -> w299
          tunnel: ["DVA OFF" ("Data Out") "DVA ON" ("Data Out")] -> w300
          frame False {
            n107 = call "WSVCAP SHL Host TL RFFE Write - Multiple DUTs - Common Data.vi"("Data Out"="074820", "error in"=w348) -> ("error out"=w347:errorcluster)  [unwired: 13 in]
          }
          frame True {
            n108 = call "WSVCAP SHL Host TL RFFE Write - Multiple DUTs - Common Data.vi"("Data Out"="074800", "error in"=w357, "Log (T)"=FALSE) -> ("error out"=w353:errorcluster)  [unwired: 12 in]
            n109 = case shown="2" "CP with DVA ON" {
              selector: "CP with DVA ON" -> [w363 w368 w373 w378 w382]
              tunnel: string[] ["07442F", "074436", "074428", "074429", "07443B"] -> [w364 w369 w374 w379 w384]
              tunnel: [w362 w367 w372 w377 w383] -> w349
              tunnel: ["35.0" ("Data Out") "29.75" ("Data Out") "30.5" ("Data Out") "44.0" ("Data Out") "40.25" ("Data Out")] -> _
              tunnel: w353 -> [w360 w365 w370 w375 w380]
              tunnel: [w360 w365 w370 w375 w380] -> w352
              frame 0, Default {
                n110 = Index Array(array=w364, index=w363) -> (element=w362:string)
              }
              frame 2 {
                n111 = Index Array(array=w369, index=w368) -> (element=w367:string)
              }
              frame 3 {
                n112 = Index Array(array=w374, index=w373) -> (element=w372:string)
              }
              frame 4 {
                n113 = Index Array(array=w379, index=w378) -> (element=w377:string)
              }
              frame 1 {
                n114 = Index Array(array=w384, index=w382) -> (element=w383:string)
              }
            }
            n115 = call "WSVCAP SHL Host TL RFFE Write - Multiple DUTs - Common Data.vi"("Data Out"=w349, "error in"=w352, "Log (T)"=FALSE) -> ("error out"=w355:errorcluster)  [unwired: 12 in]
          }
        }
        n116 = for {
          N: 36 -> [_]
          tunnel: "Serial Number" -> [w330]
          tunnel: [w328] -> w280 mode=indexing
          i -> [w327]
          n117 = Increment(x=w327) -> (x+1=w326:i32)
          n118 = Index Array(array=w330, index (row)=w326, index (col)=1 ("disabled index (col)")) -> (element=w328:string)
        }
        n119 = Not(x=w272) -> (.not. x?=w279:bool)
        n120 = Number To Fractional String(number="Set VDD", precision (6)=i16 2) -> (F-format string=w297:string)  [unwired: 2 in]
        n121 = call "Delay T4.vi"("milliseconds to wait"=w283, "error in (no error)"=w299) -> ("error out"=w287:errorcluster)  [unwired: 9 in]
        n122 = case shown="True" w276 {
          tunnel: w287 -> [w334 w336]
          tunnel: [w331 w335] -> w286
          tunnel: ["CAL OFF" ("Data Out") "CAL ON" ("Data Out")] -> w288
          frame False {
            n123 = call "WSVCAP SHL Host TL RFFE Write - Multiple DUTs - Common Data.vi"("Data Out"="074044", "error in"=w334) -> ("error out"=w331:errorcluster)  [unwired: 13 in]
          }
          frame True {
            n124 = for {
              tunnel: string[] ["074900", "074920", "074900"] -> [w344] mode=indexing
              tunnel: w336 -> [w341]
              tunnel: [w340] -> w335
              n125 = call "WSVCAP SHL Host TL RFFE Write - Multiple DUTs - Common Data.vi"("Data Out"=w344, "error in"=w341, "Log (T)"=FALSE) -> ("error out"=w343:errorcluster)  [unwired: 12 in]
              n126 = call "Delay T4.vi"("milliseconds to wait"=u32 10, "error in (no error)"=w343) -> ("error out"=w340:errorcluster)  [unwired: 9 in]
            }
          }
        }
        n127 = for {
          N: w306 -> [_]
          tunnel: w325 -> [w424]
          tunnel: [w420] -> w321
          tunnel: w294 -> [w419]
          tunnel: w314 -> [w418]
          tunnel: "TMN DC\\CAP Data Log File Path" -> [w417]
          tunnel: w312 -> [w415]
          tunnel: [w414] -> w310
          tunnel: w307 -> [w389]
          shift-right: [w409] -> _
          shift-left: u64 0 -> [w411]
          tunnel: w277 -> [w408]
          tunnel: w303 -> [w403]
          tunnel: w303 -> [w402]
          tunnel: w300 -> [w401]
          tunnel: w297 -> [w400]
          tunnel: [w399] -> w291
          tunnel: w288 -> [w398]
          tunnel: w286 -> [w397]
          tunnel: w275 -> [w396]
          tunnel: w278 -> [w394]
          tunnel: w274 -> [w393]
          tunnel: w279 -> [w392]
          tunnel: w273 -> [w391]
          tunnel: w280 -> [w390]
          tunnel: [w389] -> w269
          tunnel: w266 -> [w388]
          tunnel: w265 -> [w387]
          i -> [w407]
          stop <- w395 stop-if-true
          n128 = while {
            tunnel: w424 -> [w650]
            tunnel: w417 -> [w661]
            tunnel: "Lot#" -> [w660]
            tunnel: "Wafer#" -> [w659]
            tunnel: w390 -> [w658]
            tunnel: "Test Program" -> [w657]
            tunnel: w390 -> [w656]
            tunnel: "Comment" -> [w655]
            tunnel: "Lot#" -> [w654]
            tunnel: "Wafer#" -> [w653]
            tunnel: w418 -> [w649]
            tunnel: [w652] -> w420
            tunnel: w419 -> [w648]
            tunnel: w415 -> [w645]
            tunnel: [w644] -> w414
            tunnel: [w552] -> w405
            tunnel: w407 -> [w590]
            tunnel: [w581] -> w409
            tunnel: w411 -> [w580]
            shift-right: [w579] -> _
            shift-left: u64 0 -> [w473]
            tunnel: [w578] -> w404
            tunnel: w408 -> [w576]
            tunnel: w403 -> [w551]
            tunnel: w402 -> [w549]
            tunnel: w401 -> [w497]
            tunnel: w400 -> [w495]
            tunnel: [w470] -> w399
            tunnel: w398 -> [w477]
            tunnel: w397 -> [w476]
            tunnel: w396 -> [w475]
            tunnel: w394 -> [w467]
            tunnel: w393 -> [w466]
            tunnel: w392 -> [w461]
            tunnel: w391 -> [w455]
            tunnel: w388 -> [w431]
            tunnel: w387 -> [w430]
            i -> [w577]
            stop <- w591 stop-if-true
            n129 = case shown="4" "CP to HD/Cycle" {
              selector: "CP to HD/Cycle" -> [w665 w670 w675 w680 w684]
              tunnel: string[] ["07476F", "074776", "074765", "074769", "07477B"] -> [w666 w671 w676 w681 w686]
              tunnel: [w664 w669 w674 w679 w685] -> w492
              tunnel: ["35.0" ("Data Out") "27.5" ("Data Out") "30.5" ("Data Out") "44.0" ("Data Out") "40.25" ("Data Out")] -> w491
              tunnel: [w662 w667 w672 w677 w682] -> w490
              tunnel: w476 -> [w662 w667 w672 w677 w682]
              frame 0, Default {
                n130 = Index Array(array=w666, index=w665) -> (element=w664:string)
              }
              frame 2 {
                n131 = Index Array(array=w671, index=w670) -> (element=w669:string)
              }
              frame 3 {
                n132 = Index Array(array=w676, index=w675) -> (element=w674:string)
              }
              frame 4 {
                n133 = Index Array(array=w681, index=w680) -> (element=w679:string)
              }
              frame 1 {
                n134 = Index Array(array=w686, index=w684) -> (element=w685:string)
              }
            }
            n135 = flat-sequence {
              tunnel: [w756] -> w643
              tunnel: [w751] -> w642
              tunnel: w650 -> [w754]
              tunnel: [w753] -> w641
              tunnel: w649 -> [w731]
              tunnel: w648 -> [w752]
              tunnel: [w752] -> w640
              tunnel: [w699] -> w639
              tunnel: [w696] -> w638
              tunnel: w490 -> [w744]
              tunnel: w590 -> [w749]
              tunnel: w577 -> [w723]
              tunnel: [w723] -> w587
              tunnel: w577 -> [w748]
              tunnel: w576 -> [w746]
              tunnel: [w745] -> w575
              tunnel: [w705] -> w570
              tunnel: [w704] -> w569
              tunnel: [w703] -> w568
              tunnel: [w709] -> w558
              tunnel: [w706] -> w557
              tunnel: w551 -> [w743]
              tunnel: [w743] -> w550
              tunnel: w549 -> [w742]
              tunnel: [w708] -> w536
              tunnel: [w707] -> w510
              tunnel: [w741] -> w498
              tunnel: w492 -> [w739]
              tunnel: [w725] -> w489
              tunnel: [w724] -> w481
              tunnel: w467 -> [w719]
              tunnel: w466 -> [w718]
              tunnel: [w718] -> w465
              tunnel: w461 -> [w717]
              tunnel: [w717] -> w460
              tunnel: w455 -> [w716]
              tunnel: [w716] -> w454
              tunnel: [w711] -> w449
              tunnel: ["Test Seq"] -> w445
              tunnel: "Real No. From\nLookup Table" -> [w702]
              tunnel: ["WS1050/51"] -> w439
              tunnel: ["Cmin/Act"] -> w435
              tunnel: w431 -> [w691]
              tunnel: w430 -> [w690]
              tunnel: [w689] -> w429
              tunnel: [w687] -> w425
              tunnel: w643 -> [w1076]
              tunnel: [w1072] -> w548
              tunnel: w642 -> [w1075]
              tunnel: w641 -> [w1081]
              tunnel: [w1081] -> w547
              tunnel: w640 -> [w1080]
              tunnel: w639 -> [w1074]
              tunnel: w638 -> [w1073]
              tunnel: [w1063] -> w546
              tunnel: [w1080] -> w545
              tunnel: [w1074] -> w544
              tunnel: [w1073] -> w543
              tunnel: w587 -> [w1078]
              tunnel: [w1078] -> w542
              tunnel: w575 -> [w1077]
              tunnel: [w1077] -> w541
              tunnel: [w1075] -> w540
              tunnel: w570 -> [w1071]
              tunnel: w569 -> [w1056]
              tunnel: w568 -> [w1057]
              tunnel: [w1068] -> w539
              tunnel: w558 -> [w1070]
              tunnel: w557 -> [w1068]
              tunnel: [w1064] -> w538
              tunnel: w550 -> [w1069]
              tunnel: [w1054] -> w537
              tunnel: w536 -> [w1054]
              tunnel: [w1056] -> w535
              tunnel: w510 -> [w1055]
              tunnel: [w1055] -> w509
              tunnel: [w1057] -> w507
              tunnel: w498 -> [w1067]
              tunnel: [w1066] -> w482
              tunnel: w481 -> [w1066]
              tunnel: w465 -> [w1062]
              tunnel: [w1062] -> w464
              tunnel: w460 -> [w1061]
              tunnel: [w1061] -> w459
              tunnel: w454 -> [w1060]
              tunnel: [w1060] -> w453
              tunnel: w449 -> [w1059]
              tunnel: [w1058] -> w448
              tunnel: w445 -> [w1052]
              tunnel: [w1052] -> w444
              tunnel: w439 -> [w1051]
              tunnel: [w1051] -> w438
              tunnel: w435 -> [w1050]
              tunnel: [w1050] -> w434
              tunnel: w429 -> [w1049]
              tunnel: [w1048] -> w428
              tunnel: [w1047] -> w427
              tunnel: w425 -> [w1045]
              tunnel: w548 -> [w1243]
              tunnel: [w1242] -> w534
              tunnel: w547 -> [w1254]
              tunnel: [w1254] -> w531
              tunnel: w546 -> [w1234]
              tunnel: [w1234] -> w529
              tunnel: w545 -> [w1253]
              tunnel: [w1253] -> w527
              tunnel: w544 -> [w1252]
              tunnel: [w1252] -> w525
              tunnel: w543 -> [w1251]
              tunnel: [w1251] -> w523
              tunnel: w542 -> [w1250]
              tunnel: [w1250] -> w521
              tunnel: w541 -> [w1249]
              tunnel: [w1249] -> w519
              tunnel: w540 -> [w1248]
              tunnel: [w1248] -> w517
              tunnel: w539 -> [w1247]
              tunnel: [w1247] -> w515
              tunnel: [w1239] -> w513
              tunnel: w538 -> [w1238]
              tunnel: w537 -> [w1245]
              tunnel: w535 -> [w1244]
              tunnel: w509 -> [w1231]
              tunnel: [w1231] -> w508
              tunnel: w507 -> [w1233]
              tunnel: [w1233] -> w506
              tunnel: [w1240] -> w505
              tunnel: [w1241] -> w483
              tunnel: w482 -> [w1241]
              tunnel: w464 -> [w1237]
              tunnel: [w1237] -> w463
              tunnel: w459 -> [w1236]
              tunnel: [w1236] -> w458
              tunnel: w453 -> [w1235]
              tunnel: [w1235] -> w452
              tunnel: w448 -> [w1232]
              tunnel: w444 -> [w1229]
              tunnel: [w1232] -> w443
              tunnel: [w1229] -> w442
              tunnel: w438 -> [w1228]
              tunnel: [w1228] -> w437
              tunnel: w434 -> [w1227]
              tunnel: [w1227] -> w433
              tunnel: w428 -> [w1226]
              tunnel: w427 -> [w1225]
              tunnel: [w1224] -> w426
              tunnel: w534 -> [w1342]
              tunnel: [w1341] -> w533
              tunnel: [w1337] -> w532
              tunnel: w531 -> [w1354]
              tunnel: [w1354] -> w530
              tunnel: w529 -> [w1331]
              tunnel: [w1331] -> w528
              tunnel: w527 -> [w1353]
              tunnel: [w1353] -> w526
              tunnel: w525 -> [w1352]
              tunnel: [w1352] -> w524
              tunnel: w523 -> [w1351]
              tunnel: [w1351] -> w522
              tunnel: w521 -> [w1350]
              tunnel: [w1350] -> w520
              tunnel: w519 -> [w1349]
              tunnel: [w1349] -> w518
              tunnel: w517 -> [w1348]
              tunnel: [w1348] -> w516
              tunnel: w515 -> [w1347]
              tunnel: [w1347] -> w514
              tunnel: w513 -> [w1346]
              tunnel: [w1346] -> w512
              tunnel: [w1328] -> w511
              tunnel: w508 -> [w1344]
              tunnel: w506 -> [w1343]
              tunnel: w505 -> [w1336]
              tunnel: ["DeltaC Target Setting(pF)"] -> w496
              tunnel: [w1339] -> w484
              tunnel: w483 -> [w1339]
              tunnel: w475 -> [w1338]
              tunnel: [w1338] -> w474
              tunnel: w463 -> [w1335]
              tunnel: [w1335] -> w462
              tunnel: w458 -> [w1334]
              tunnel: [w1334] -> w457
              tunnel: w452 -> [w1333]
              tunnel: [w1333] -> w451
              tunnel: w443 -> [w1332]
              tunnel: w442 -> [w1329]
              tunnel: [w1328] -> w440
              tunnel: w437 -> [w1327]
              tunnel: [w1327] -> w436
              tunnel: w433 -> [w1326]
              tunnel: [w1326] -> w432
              tunnel: w426 -> [w1325]
              tunnel: [w1473] -> w637
              tunnel: [w1440] -> w636
              tunnel: w533 -> [w1475]
              tunnel: w532 -> [w1454]
              tunnel: [w1463] -> w635
              tunnel: [w1454] -> w634
              tunnel: [w1424] -> w633
              tunnel: [w1422] -> w632
              tunnel: w530 -> [w1474]
              tunnel: [w1474] -> w631
              tunnel: w528 -> [w1463]
              tunnel: w526 -> [w1472]
              tunnel: [w1472] -> w630
              tunnel: w524 -> [w1468]
              tunnel: [w1468] -> w629
              tunnel: w522 -> [w1467]
              tunnel: [w1467] -> w628
              tunnel: w520 -> [w1464]
              tunnel: [w1464] -> w586
              tunnel: w518 -> [w1471]
              tunnel: [w1471] -> w574
              tunnel: w516 -> [w1470]
              tunnel: [w1469] -> w571
              tunnel: w514 -> [w1466]
              tunnel: w512 -> [w1462]
              tunnel: [w1423] -> w567
              tunnel: [w1465] -> w566
              tunnel: [w1462] -> w561
              tunnel: w511 -> [w1461]
              tunnel: [w1448] -> w556
              tunnel: [w1447] -> w555
              tunnel: [w1446] -> w554
              tunnel: w496 -> [w1460]
              tunnel: [w1445] -> w485
              tunnel: w484 -> [w1445]
              tunnel: [w1444] -> w480
              tunnel: w474 -> [w1443]
              tunnel: w462 -> [w1438]
              tunnel: w457 -> [w1437]
              tunnel: [w1437] -> w456
              tunnel: w451 -> [w1436]
              tunnel: [w1436] -> w450
              tunnel: w440 -> [w1433]
              tunnel: w436 -> [w1432]
              tunnel: w432 -> [w1427]
              tunnel: w637 -> [w1629]
              tunnel: [w1629] -> w627
              tunnel: [w1614] -> w626
              tunnel: [w1628] -> w625
              tunnel: w636 -> [w1627]
              tunnel: w635 -> [w1626]
              tunnel: w634 -> [w1625]
              tunnel: [w1626] -> w624
              tunnel: [w1625] -> w623
              tunnel: w633 -> [w1624]
              tunnel: [w1624] -> w622
              tunnel: w632 -> [w1623]
              tunnel: [w1623] -> w621
              tunnel: w631 -> [w1622]
              tunnel: [w1622] -> w620
              tunnel: w630 -> [w1621]
              tunnel: [w1621] -> w619
              tunnel: w629 -> [w1620]
              tunnel: [w1620] -> w618
              tunnel: w628 -> [w1619]
              tunnel: [w1619] -> w617
              tunnel: w645 -> [w1618]
              tunnel: [w1616] -> w616
              tunnel: [w1596] -> w615
              tunnel: [w1597] -> w614
              tunnel: [w1595] -> w613
              tunnel: w586 -> [w1612]
              tunnel: [w1612] -> w585
              tunnel: w574 -> [w1611]
              tunnel: [w1611] -> w573
              tunnel: w571 -> [w1628]
              tunnel: w567 -> [w1609]
              tunnel: w566 -> [w1610]
              tunnel: [w1610] -> w565
              tunnel: [w1609] -> w563
              tunnel: w561 -> [w1608]
              tunnel: [w1608] -> w560
              tunnel: w556 -> [w1594]
              tunnel: w555 -> [w1593]
              tunnel: w554 -> [w1592]
              tunnel: [w1589] -> w553
              tunnel: [w1594] -> w504
              tunnel: [w1593] -> w502
              tunnel: [w1592] -> w500
              tunnel: [w1591] -> w486
              tunnel: w485 -> [w1591]
              tunnel: w480 -> [w1590]
              tunnel: [w1590] -> w479
              tunnel: w456 -> [w1589]
              tunnel: w450 -> [w1588]
              tunnel: w627 -> [w1714]
              tunnel: [w1714] -> w612
              tunnel: w626 -> [w1738]
              tunnel: [w1737] -> w611
              tunnel: w661 -> [w1739]
              tunnel: w660 -> [w1736]
              tunnel: w659 -> [w1735]
              tunnel: w658 -> [w1734]
              tunnel: [w1733] -> w610
              tunnel: w625 -> [w1727]
              tunnel: [w1727] -> w609
              tunnel: w624 -> [w1732]
              tunnel: w623 -> [w1731]
              tunnel: [w1732] -> w608
              tunnel: [w1731] -> w607
              tunnel: [w1722] -> w606
              tunnel: w622 -> [w1730]
              tunnel: [w1730] -> w605
              tunnel: w621 -> [w1729]
              tunnel: [w1729] -> w604
              tunnel: w620 -> [w1726]
              tunnel: [w1728] -> w603
              tunnel: w473 -> [w1725]
              tunnel: [w1724] -> w602
              tunnel: [w1712] -> w601
              tunnel: w619 -> [w1723]
              tunnel: w618 -> [w1721]
              tunnel: w617 -> [w1720]
              tunnel: "File Name" -> [w1719]
              tunnel: w616 -> [w1718]
              tunnel: [w1718] -> w600
              tunnel: w615 -> [w1717]
              tunnel: [w1717] -> w599
              tunnel: [w1716] -> w598
              tunnel: w614 -> [w1716]
              tunnel: w613 -> [w1715]
              tunnel: [w1715] -> w597
              tunnel: [w1710] -> w588
              tunnel: w585 -> [w1711]
              tunnel: [w1711] -> w583
              tunnel: w580 -> [w1709]
              tunnel: w573 -> [w1708]
              tunnel: [w1708] -> w572
              tunnel: w565 -> [w1707]
              tunnel: [w1707] -> w564
              tunnel: w563 -> [w1706]
              tunnel: [w1706] -> w562
              tunnel: w560 -> [w1705]
              tunnel: [w1705] -> w559
              tunnel: w553 -> [w1704]
              tunnel: w504 -> [w1703]
              tunnel: [w1703] -> w503
              tunnel: w502 -> [w1702]
              tunnel: [w1702] -> w501
              tunnel: w500 -> [w1701]
              tunnel: [w1701] -> w499
              tunnel: w489 -> [w1700]
              tunnel: [w1700] -> w488
              tunnel: [w1699] -> w487
              tunnel: w486 -> [w1699]
              tunnel: w479 -> [w1698]
              tunnel: [w1698] -> w478
              tunnel: ["Freq(Hz)"] -> w447
              tunnel: ["Board#"] -> w446
              tunnel: w612 -> [w1811]
              tunnel: w611 -> [w1810]
              tunnel: w661 -> [w1773]
              tunnel: w657 -> [w1805]
              tunnel: w656 -> [w1808]
              tunnel: w655 -> [w1804]
              tunnel: w654 -> [w1807]
              tunnel: w653 -> [w1803]
              tunnel: w610 -> [w1806]
              tunnel: [w1811] -> w593
              tunnel: [w1809] -> w594
              tunnel: w609 -> [w1801]
              tunnel: [w1801] -> w595
              tunnel: w608 -> [w1800]
              tunnel: w607 -> [w1785]
              tunnel: w606 -> [w1799]
              tunnel: w605 -> [w1798]
              tunnel: w604 -> [w1787]
              tunnel: [w1795] -> w596
              tunnel: w603 -> [w1797]
              tunnel: w602 -> [w1796]
              tunnel: w601 -> [w1795]
              tunnel: "File Name" -> [w1766]
              tunnel: w600 -> [w1794]
              tunnel: [w1794] -> w592
              tunnel: w599 -> [w1793]
              tunnel: w598 -> [w1792]
              tunnel: w597 -> [w1791]
              tunnel: [w1790] -> w589
              tunnel: w588 -> [w1790]
              tunnel: [w1769] -> w584
              tunnel: w583 -> [w1769]
              tunnel: w572 -> [w1789]
              tunnel: w564 -> [w1788]
              tunnel: w562 -> [w1786]
              tunnel: w559 -> [w1784]
              tunnel: w503 -> [w1783]
              tunnel: w501 -> [w1782]
              tunnel: w499 -> [w1781]
              tunnel: w497 -> [w1780]
              tunnel: w477 -> [w1779]
              tunnel: w491 -> [w1778]
              tunnel: w495 -> [w1777]
              tunnel: w488 -> [w1776]
              tunnel: w487 -> [w1775]
              tunnel: w478 -> [w1774]
              tunnel: [w1771] -> w472
              tunnel: [w1762] -> w468
              tunnel: w447 -> [w1761]
              tunnel: w446 -> [w1759]
              tunnel: [w1832] -> w651
              tunnel: [w1833] -> w652
              tunnel: [w1834] -> w552
              tunnel: w596 -> [w1825]
              tunnel: w595 -> [w1833]
              tunnel: w594 -> [w1820]
              tunnel: w593 -> [w1834]
              tunnel: w592 -> [w1827]
              tunnel: [w1827] -> w644
              tunnel: [w1824] -> w581
              tunnel: w589 -> [w1824]
              tunnel: w584 -> [w1826]
              tunnel: [w1826] -> w582
              tunnel: [w1825] -> w579
              tunnel: [w1823] -> w578
              tunnel: [w1819] -> w469
              tunnel: w472 -> [w1818]
              tunnel: w468 -> [w1816]
              frame #0 {
                w712 = FALSE ("Log (T)")
                n136 = call "WSVCAP SHL Host TL RFFE Write - Multiple DUTs - Common Data.vi"("Data Out"=w739, "error in"=w744, "Log (T)"=FALSE) -> ("error out"=w721:errorcluster)  [unwired: 12 in]
                n137 = Index Array(array=w754, index (row)=w748, index (col)=0 ("disabled index (col)")) -> (element=w747:dbl)
                n138 = for {
                  tunnel: string[] ["0760", "0767", "0768"] -> [w803] mode=indexing
                  tunnel: [w799] -> w729 mode=indexing
                  tunnel: w721 -> [w797]
                  tunnel: [w796] -> w722
                  i -> [w802]
                  n139 = call "Delay T4.vi"("milliseconds to wait"=u32 10, "error in (no error)"=w797) -> ("error out"=w804:errorcluster)  [unwired: 9 in]
                  n140 = call "WSVCAP SHL Host TL RFFE Read - Multiple DUTs - Common Data.vi"("Data Out"=w803, "error in"=w804, "Log (T)"=FALSE) -> ("RFFE Data In"=w801:string[], "error out"=w796:errorcluster)  [unwired: 11 in]
                  n141 = Index Array(array=w801, index=w802) -> (element=w798:string)
                  n142 = String Subset(string=w798, offset (0)=0) -> (substring=w799:string)  [unwired: 1 in]
                }
                "RB Reg for HD/Cycle" <- w729
                n143 = local read "IDD Brd(uA)"() -> (w738:string)
                n144 = call "Delay T4.vi"("milliseconds to wait"=u32 100, "error in (no error)"=w722) -> ("error out"=w734:errorcluster)  [unwired: 9 in]
                n145 = call "Ke2000 Single Reading.vi"("error in (no error)"=w734, "VISA resource name"=w731) -> ("error out"=w736:errorcluster, "VISA resource name out"=w701:refnum<visa-resource-name>, "uA"=w737:string)  [unwired: 5 in, 2 out]
                n146 = call "Substration.vi"("error in (no error)"=w736, "Input2"=w738, "Input1"=w737) -> ("error out"=w733:errorcluster, "In1 - In2"=→"IDD_HD/CYC (uA)":string)  [unwired: 7 in]
                n147 = case shown="False" w746 {
                  tunnel: [w835 w940] -> w756
                  tunnel: [w836 w925] -> w715
                  tunnel: [w834 w941] -> w753
                  tunnel: w733 -> [w830 w929]
                  tunnel: w749 -> [_ w931]
                  tunnel: w747 -> [w827 w926]
                  tunnel: [w832 w927] -> w745
                  tunnel: w723 -> [w819 w923]
                  tunnel: w742 -> [w829 _]
                  tunnel: ["% Duty Cycle" "100" ("Data Out")] -> w725
                  tunnel: w719 -> [w817 _]
                  tunnel: w702 -> [w816 w918]
                  tunnel: w691 -> [w813 _]
                  tunnel: w690 -> [w812 _]
                  frame False {
                    # "Cycles in 1s"
                    n148 = case shown="True" w816 {
                      tunnel: w830 -> [w842 w848]
                      tunnel: w827 -> [w841 w847]
                      tunnel: [w840 w848] -> w826
                      tunnel: w819 -> [w839 _]
                      tunnel: [w838 w847] -> w825
                      tunnel: [u64 1000 ("y") u64 1 ("y")] -> w820
                      frame False {
                        n149 = case shown="8, Default" w839 {
                          tunnel: w841 -> [w844 _]
                          tunnel: [w844 "Cycle RP"] -> w838
                          tunnel: [w843 w845] -> w840
                          tunnel: w842 -> [w843 w845]
                          frame 0..7 {
                          }
                          frame 8, Default {
                          }
                        }
                      }
                      frame True {
                        # "Read real number\nfrom lookup table"
                      }
                    }
                    n150 = call "WSVCAP SHL Host TL RFFE Configure.vi"("RFFE Slave Address"=w829, "Clock Rate (Hz)"="SPI Clock Rate (Hz)", "error in"=w826) -> ("Actual Rate (Hz)"=→"AR Cycling(Hz)":dbl, "error out"=w815:errorcluster)  [unwired: 11 in]
                    n151 = Array Max & Min(array=w812) -> (max value=w823:dbl)  [unwired: 3 out]
                    n152 = Divide(x=1.0, y=w823) -> (x/y=w822:dbl)
                    n153 = To Unsigned Quad Integer(1:w822) -> (0:w821:u64)
                    n154 = Not(x=w817) -> (.not. x?=w818:bool)
                    n155 = case shown="True" w818 {
                      tunnel: [w851 w873] -> w836
                      tunnel: [w854 w872] -> w835
                      tunnel: [u64 1 w871] -> w834
                      tunnel: w815 -> [w852 w870]
                      tunnel: w825 -> [_ w869]
                      tunnel: w812 -> [_ w867]
                      tunnel: w821 -> [_ w866]
                      tunnel: w820 -> [_ w865]
                      tunnel: w819 -> [w850 _]
                      tunnel: w813 -> [_ w864]
                      frame False {
                        n156 = case shown="1, Default" w850 {
                          tunnel: w852 -> [w855 w857]
                          tunnel: [w855 w856] -> w851
                          frame 0 {
                          }
                          frame 1, Default {
                            n157 = flat-sequence {
                              tunnel: "Repeat Meas(s)" -> [w863]
                              tunnel: w857 -> [w860]
                              tunnel: [w860] -> w856
                              frame #0 {
                                n158 = Multiply(x=w863, y=u32 1000) -> (x*y=w862:u32)
                                n159 = Wait (ms)(milliseconds to wait=w862) -> ()  [unwired: 1 out]
                                n160 = local write "STATUS"("Verify Sockets waiting times..." ("STATUS")) -> ()
                              }
                            }
                          }
                        }
                        n161 = local read "stop During HD/Cycles"() -> (w854:bool)
                      }
                      frame True {
                        n162 = while {
                          tunnel: w869 -> [w893]
                          tunnel: [w880] -> w873
                          tunnel: [w885] -> w872
                          tunnel: w870 -> [w891]
                          tunnel: [w879] -> w871
                          tunnel: w864 -> [w890]
                          tunnel: w867 -> [w889]
                          tunnel: w866 -> [w876]
                          tunnel: w865 -> [w874]
                          i -> [w888]
                          stop <- w884 stop-if-true
                          # "At least 1 second before target"
                          # "Remaining Cycles"
                          # "Target Cycles"
                          # "Cycles in 1s"
                          n163 = To Unsigned Quad Integer(1:w893) -> (0:w892:u64)
                          n164 = case shown="0" w888 {
                            tunnel: [w901 w903] -> w882
                            tunnel: w891 -> [w902 w903]
                            tunnel: w890 -> [w900 _]
                            tunnel: w889 -> [w899 _]
                            frame 0 {
                              n165 = call "WSVCAP SHL Host TL RFFE Write Cycle - Multiple DUTs - Common Data.vi"("Data Out (Cycle Commands)"=w900, "Post Command Delay"=w899, "error in"=w902, "Log (T)"=FALSE) -> ("error out"=w901:errorcluster)  [unwired: 11 in]
                            }
                            frame 1, Default {
                            }
                          }
                          n166 = Multiply(x=w892, y=w874) -> (x*y=w879:u64)
                          n167 = call "WSVCAP SHL Host TL SPI_RFFE Query Cycle Count.vi"("error in"=w882) -> ("Cycle Count"=w878:u64, "error out"=w887:errorcluster)  [unwired: 13 in]
                          "Cycle Count" <- w878
                          n168 = Subtract(x=w879, y=w878) -> (x-y=w877:u64)
                          n169 = Greater Or Equal?(x=w878, y=w879) -> (x >= y?=w886:bool)
                          n170 = local read "stop During HD/Cycles"() -> (w885:bool)
                          n171 = Greater?(x=w877, y=w876) -> (0:w875:bool)
                          n172 = case shown="True" w886 {
                            tunnel: [w905 w908] -> w881
                            tunnel: w887 -> [w905 w907]
                            tunnel: [FALSE TRUE] -> w883
                            frame False {
                            }
                            frame True {
                              n173 = call "WSVCAP SHL Host TL SPI Stop Write Cycle.vi"("error in"=w907) -> ("error out"=w908:errorcluster)  [unwired: 14 in]
                            }
                          }
                          n174 = Or(x=w883, y=w885) -> (x .or. y?=w884:bool)
                          n175 = case shown="True" w875 {
                            tunnel: w881 -> [w894 w897]
                            tunnel: [w894 w896] -> w880
                            frame False {
                            }
                            frame True {
                              n176 = call "MISC Wait with Data Flow.vi"("Error In (no error)"=w897, "Wait Time (500ms)"=u32 50) -> ("Error Out"=w896:errorcluster)  [unwired: 7 in, 2 out]
                            }
                          }
                        }
                        n177 = local write "STATUS"("Parts are Cycling...." ("STATUS")) -> ()
                      }
                    }
                    n178 = local read "HD/CYC Temp"() -> (w831:i32)
                    n179 = Number To Engineering String(4:w831) -> (0:w832:string)  [unwired: 3 in]
                  }
                  frame True {
                    n180 = case shown="False" w918 {
                      tunnel: w931 -> [w958 _]
                      tunnel: [w957 w970] -> w930
                      tunnel: w929 -> [w956 w971]
                      tunnel: [w955 w971] -> w928
                      tunnel: w926 -> [w954 w970]
                      tunnel: w923 -> [w953 _]
                      frame False {
                        n181 = case shown="1, Default" w958 {
                          tunnel: [w961 w968] -> w957
                          tunnel: w956 -> [w963 w969]
                          tunnel: [w962 w969] -> w955
                          tunnel: w954 -> [w960 _]
                          tunnel: w953 -> [w959 _]
                          frame 0 {
                            n182 = case shown="15, Default" w959 {
                              tunnel: [w964 "HD RP"] -> w961
                              tunnel: w963 -> [w965 w966]
                              tunnel: [w965 w966] -> w962
                              tunnel: w960 -> [w964 _]
                              frame 0..14 {
                              }
                              frame 15, Default {
                              }
                            }
                          }
                          frame 1, Default {
                            n183 = local read "HD RP"() -> (w968:dbl)
                          }
                        }
                      }
                      frame True {
                      }
                    }
                    n184 = call "WSVCAP SHL Host TL RFFE Write - Multiple DUTs - Common Data.vi"("Data Out"="Cmd To HD", "error in"=w928, "Log (T)"=FALSE) -> ("error out"=w914:errorcluster)  [unwired: 12 in]
                    n185 = local read "No of HD/Cycle\nCompleted"() -> (w932:u64)
                    n186 = call "Delay T4.vi"("milliseconds to wait"=u32 50, "error in (no error)"=w914) -> ("error out"=w911:errorcluster)  [unwired: 9 in]
                    n187 = for {
                      tunnel: string[] ["0761", "0762", "0763"] -> [w952] mode=indexing
                      tunnel: [w948] -> w910 mode=indexing
                      shift-right: [w945] -> w936
                      shift-left: w911 -> [w951]
                      i -> [w950]
                      n188 = call "WSVCAP SHL Host TL RFFE Read - Multiple DUTs - Common Data.vi"("Data Out"=w952, "error in"=w951, "Log (T)"=FALSE) -> ("RFFE Data In"=w947:string[], "error out"=w944:errorcluster)  [unwired: 11 in]
                      n189 = Index Array(array=w947, index=w950) -> (element=w946:string)
                      n190 = call "Delay T4.vi"("milliseconds to wait"=u32 10, "error in (no error)"=w944) -> ("error out"=w945:errorcluster)  [unwired: 9 in]
                      n191 = String Subset(string=w946, offset (0)=0) -> (substring=w948:string)  [unwired: 1 in]
                    }
                    "RB Reg for HD" <- w910
                    n192 = Greater?(x="HD_DC (Min)", y=w932) -> (0:w933:bool)
                    n193 = case shown="True" w933 {
                      tunnel: [_ w982] -> w938
                      tunnel: [w973 w981] -> w937
                      tunnel: w936 -> [w973 w980]
                      tunnel: w930 -> [w972 w979]
                      tunnel: [w972 w979] -> w935
                      frame False {
                      }
                      frame True {
                        n194 = Multiply(x=1000.0, y=w979) -> (x*y=w977:dbl)
                        n195 = Multiply(x=60.0, y=w977) -> (x*y=w975:dbl)
                        n196 = local write "STATUS"("Parts are Holding Down..." ("STATUS")) -> ()
                        n197 = event shown="[0] Timeout" {
                          selector: _ -> [_ _]
                          dyn-events: _ -> [_ _]
                          timeout: w975 -> [_ _]
                          tunnel: ["stop During HD/Cycles" TRUE ("stop During HD/Cycles")] -> w982
                          tunnel: w980 -> [w983 w985]
                          tunnel: [w983 w985] -> w981
                          event Timeout {
                            n198 = event-data() -> ()  [unwired: 1 in, 2 out]
                          }
                          event "stop During HD/Cycles": Value Change {
                            n199 = event-data() -> ()  [unwired: 1 in, 2 out]
                          }
                        }
                      }
                    }
                    n200 = Greater Or Equal?(x=w932, y="HD_DC (Min)") -> (x >= y?=w939:bool)
                    n201 = To Unsigned Quad Integer(1:w930) -> (0:w941:u64)
                    n202 = Add(x="Time All OFF (s)", y="Time All ON (s)") -> (x+y=w920:u32)
                    n203 = To Double Precision Float(number=w920) -> (double precision float=w919:dbl)
                    n204 = Divide(x=w919, y=60.0) -> (x/y=w921:dbl)
                    n205 = case shown="False" w939 {
                      tunnel: [w989 w1005] -> w940
                      tunnel: [w990 w997] -> w925
                      tunnel: w937 -> [w990 w1004]
                      tunnel: w938 -> [w989 w1003]
                      tunnel: w935 -> [_ w1002]
                      tunnel: [w988 w1000] -> w927
                      tunnel: w921 -> [_ w994]
                      tunnel: "Time All OFF (s)" -> [_ w992]
                      tunnel: "Time All ON (s)" -> [_ w991]
                      frame False {
                        n206 = Number To Engineering String(4:"HD/CYC Temp") -> (0:w988:string)  [unwired: 3 in]
                      }
                      frame True {
                        n207 = Divide(x=w1002, y=w994) -> (x/y=w1001:dbl)
                        n208 = call "WSVCAP SHL Host TL RFFE Write - Multiple DUTs - Common Data.vi"("Data Out"="070201000000", "error in"=w1004, "Log (T)"=FALSE) -> ("error out"=w1007:errorcluster)  [unwired: 12 in]
                        n209 = Round To Nearest(number=w1001) -> (nearest integer value=w996:dbl)
                        n210 = call "Delay T4.vi"("milliseconds to wait"=u32 50, "error in (no error)"=w1007) -> ("error out"=w998:errorcluster)  [unwired: 9 in]
                        n211 = To Long Integer(number=w996) -> (32bit integer=w995:i32)
                        "No LPs to RP" <- w995
                        n212 = for {
                          N: w995 -> [_]
                          tunnel: w1003 -> [w1025]
                          tunnel: [w1024] -> w1005
                          tunnel: w998 -> [w1014]
                          tunnel: [w1013] -> w997
                          tunnel: w992 -> [w1011]
                          tunnel: w991 -> [w1009]
                          i -> [w1023]
                          stop <- w1024 stop-if-true
                          w1012 = FALSE ("Log (T)")
                          w1010 = u32 1 ("milliseconds to wait")
                          n213 = Increment(x=w1023) -> (x+1=→"LPs Count":i32)
                          n214 = call "WSVCAP SHL Host TL RFFE Write - Multiple DUTs - Common Data.vi"("Data Out"="074776", "error in"=w1014, "Log (T)"=w1012) -> ("error out"=w1031:errorcluster)  [unwired: 12 in]
                          n215 = call "Delay T4.vi"("milliseconds to wait"=w1010, "error in (no error)"=w1031) -> ("error out"=w1030:errorcluster)  [unwired: 9 in]
                          n216 = local read "CP to HD/Cycle"() -> (w1016:i32)
                          n217 = call "WSVCAP SHL Host TL RFFE Write - Multiple DUTs - Common Data.vi"("Data Out"="070201000000", "error in"=w1017) -> ("error out"=w1027:errorcluster)  [unwired: 13 in]
                          n218 = call "WSVCAP SHL Host TL RFFE Write - Multiple DUTs - Common Data.vi"("Data Out"="0702013B3B3B", "error in"=w1030, "Log (T)"=w1012) -> ("error out"=w1020:errorcluster)  [unwired: 12 in]
                          n219 = call "Delay T4.vi"("milliseconds to wait"=w1010, "error in (no error)"=w1020) -> ("error out"=w1019:errorcluster)  [unwired: 9 in]
                          n220 = flat-sequence {
                            tunnel: w1027 -> [w1038]
                            tunnel: [w1036] -> w1013
                            tunnel: w1011 -> [w1033]
                            frame #0 {
                              n221 = local write "STATUS"("Now HD OFF Time..." ("STATUS")) -> ()
                              n222 = Multiply(x=w1033, y=u32 1000) -> (x*y=w1035:u32)
                              n223 = call "Delay T4.vi"("milliseconds to wait"=w1035, "error in (no error)"=w1038) -> ("error out"=w1036:errorcluster)  [unwired: 9 in]
                            }
                          }
                          n224 = Index Array(array=string[] ["07476F", "074776", "074765", "074769", "07477B"], index=w1016) -> (element=w1021:string)
                          n225 = call "WSVCAP SHL Host TL RFFE Write - Multiple DUTs - Common Data.vi"("Data Out"=w1021, "error in"=w1019, "Log (T)"=w1012) -> ("error out"=w1018:errorcluster)  [unwired: 12 in]
                          n226 = flat-sequence {
                            tunnel: [w1043] -> w1017
                            tunnel: w1018 -> [w1040]
                            tunnel: w1009 -> [w1039]
                            frame #0 {
                              n227 = local write "STATUS"("Now HD ON Time..." ("STATUS")) -> ()
                              n228 = Multiply(x=w1039, y=u32 1000) -> (x*y=w1042:u32)
                              n229 = call "Delay T4.vi"("milliseconds to wait"=w1042, "error in (no error)"=w1040) -> ("error out"=w1043:errorcluster)  [unwired: 9 in]
                            }
                          }
                          n230 = Unbundle By Name(w1013) -> ("status"=w1026:bool)
                          n231 = Or(x=w1026, y=w1025) -> (x .or. y?=w1024:bool)
                        }
                        n232 = Number To Engineering String(4:"DC_Temp") -> (0:w1000:string)  [unwired: 3 in]
                      }
                    }
                  }
                }
                n233 = case shown="0, Default" "CP to Meas" {
                  selector: "CP to Meas" -> [w773 w778 w783 w788 w792]
                  tunnel: string[] ["07476F", "074776", "074765", "074769", "07477B"] -> [w774 w779 w784 w789 w794]
                  tunnel: [w772 w777 w782 w787 w793] -> w727
                  tunnel: [w771 w776 w781 w786 w791] -> w720
                  tunnel: w715 -> [w771 w776 w781 w786 w791]
                  tunnel: ["35.0" ("Data Out") "27.5" ("Data Out") "30.5" ("Data Out") "44.0" ("Data Out") "40.25" ("Data Out")] -> w724
                  frame 0, Default {
                    n234 = Index Array(array=w774, index=w773) -> (element=w772:string)
                  }
                  frame 2 {
                    n235 = Index Array(array=w779, index=w778) -> (element=w777:string)
                  }
                  frame 3 {
                    n236 = Index Array(array=w784, index=w783) -> (element=w782:string)
                  }
                  frame 4 {
                    n237 = Index Array(array=w789, index=w788) -> (element=w787:string)
                  }
                  frame 1 {
                    n238 = Index Array(array=w794, index=w792) -> (element=w793:string)
                  }
                }
                n239 = call "WSVCAP SHL Host TL RFFE Write - Multiple DUTs - Common Data.vi"("Data Out"=w727, "error in"=w720, "Log (T)"=w712) -> ("error out"=w740:errorcluster)  [unwired: 12 in]
                n240 = flat-sequence {
                  tunnel: w714 -> [w806]
                  tunnel: [w806] -> w710
                  frame #0 {
                    w808 = "0" ("NOM IDD OFF(uA)")
                    w809 = string[] []
                    w810 = string[][] []
                    n241 = To Long Integer(number=0.0 ("No of Loops to RP")) -> (32bit integer=w807:i32)
                    n242 = local write "NOM IDD ON (uA)"(w808) -> ()
                    n243 = local write "Total Delta C1(pF)"(w809) -> ()
                    n244 = local write "Total Delta C2(pF)"(w809) -> ()
                    n245 = local write "Total Delta C3(pF)"(w809) -> ()
                    n246 = local write "Current EFuse Read back"(w809) -> ()
                    n247 = local write "RB Reg for HD"(w809) -> ()
                    n248 = local write "RB Reg for HD/Cycle"(w809) -> ()
                    n249 = local write "NOM IDD OFF(uA)"(w808) -> ()
                    n250 = local write "LPs Count"(w807) -> ()
                    n251 = local write "No LPs to RP"(w807) -> ()
                    n252 = local write "VSA_V3"(w810) -> ()
                    n253 = local write "VSA_V1"(w810) -> ()
                    n254 = local write "VSA_V2"(w810) -> ()
                    n255 = local write "VPI C1"(w810) -> ()
                    n256 = local write "VPI C2"(w810) -> ()
                    n257 = local write "VPI C3"(w810) -> ()
                    n258 = local write "% Delta C"(w810) -> ()
                    n259 = local write "40V_3"(w810) -> ()
                    n260 = local write "40V_2"(w810) -> ()
                    n261 = local write "40V_1"(w810) -> ()
                  }
                }
                n262 = call "Delay T4.vi"("milliseconds to wait"=u32 50, "error in (no error)"=w740) -> ("error out"=w694:errorcluster)  [unwired: 9 in]
                n263 = for {
                  tunnel: [w769] -> w751
                  tunnel: [w768] -> w714
                  tunnel: w712 -> [w767]
                  tunnel: w701 -> [w766]
                  tunnel: w694 -> [w762]
                  tunnel: string[] ["0702013B3B3B", "070201000000"] -> [w758] mode=indexing
                  tunnel: [w757] -> w697 mode=indexing
                  n264 = call "WSVCAP SHL Host TL RFFE Write - Multiple DUTs - Common Data.vi"("Data Out"=w758, "error in"=w762, "Log (T)"=w767) -> ("error out"=w763:errorcluster)  [unwired: 12 in]
                  n265 = local read "IDD Brd(uA)"() -> (w759:string)
                  n266 = call "Delay T4.vi"("milliseconds to wait"=u32 100, "error in (no error)"=w763) -> ("error out"=w764:errorcluster)  [unwired: 9 in]
                  n267 = call "Ke2000 Single Reading.vi"("error in (no error)"=w764, "VISA resource name"=w766) -> ("error out"=w761:errorcluster, "VISA resource name out"=w769:refnum<visa-resource-name>, "uA"=w760:string)  [unwired: 5 in, 2 out]
                  n268 = call "Substration.vi"("error in (no error)"=w761, "Input2"=w759, "Input1"=w760) -> ("error out"=w768:errorcluster, "In1 - In2"=w757:string)  [unwired: 7 in]
                }
                n269 = Index Array(array=w697, index=1) -> (element=w696:string)
                n270 = Index Array(array=w697, index=0) -> (element=w699:string)
                n271 = local read "Clock Rate (Hz)"() -> (w741:dbl)
                n272 = call "Multi Dut Cmd_Header Setting.vi"("WS1050/51"="WS1050/51", "Cmin/Act"="Cmin/Act", "Test Seq"="Test Seq", "error in (no error)"=w710) -> ("Name 1"=w709:string[], "Name_ALL"=w687:string[], "Name 2"=w708:string[], "Name Header"=w706:string[], "Name 3"=w707:string[], "Cmd 3"=w703:string[], "Cmd 1"=w705:string[], "Extended Cmd"=w689:string[], "Cmd 2"=w704:string[], "error out"=w711:errorcluster)  [unwired: 2 in]
              }
              frame #1 {
                w1058 = FALSE ("Log (T)")
                n273 = call "WSVCAP SHL Host TL RFFE Configure.vi"("RFFE Slave Address"=w1069, "Clock Rate (Hz)"=w1067, "error in"=w1059) -> ("Actual Rate (Hz)"=w1079:dbl, "error out"=w1065:errorcluster)  [unwired: 11 in]
                n274 = local write "AR  Measurent(Hz)"(w1079) -> ()
                n275 = Array Size(array=w1070) -> (size(s)=w1082:i32)
                n276 = case shown="3" w1052 {
                  tunnel: w1082 -> [w1092 w1125 w1158 w1192]
                  tunnel: w1076 -> [w1091 w1124 w1157 w1191]
                  tunnel: [w1090 w1123 w1156 w1190] -> w1072
                  tunnel: w1071 -> [w1089 w1122 w1155 _]
                  tunnel: w1070 -> [w1088 w1121 w1154 _]
                  tunnel: w1065 -> [w1087 w1120 w1153 w1189]
                  tunnel: [w1086 w1119 w1152 w1188] -> w1064
                  tunnel: w1058 -> [w1085 w1118 w1151 w1187]
                  tunnel: [w1084 w1117 w1150 w1186] -> w1053
                  tunnel: w1049 -> [_ _ _ w1183]
                  tunnel: [w1083 w1116 w1149 w1185] -> w1048
                  tunnel: [w1083 w1116 w1149 w1184] -> w1047
                  tunnel: string[][] [] -> [w1083 w1116 w1149 _]
                  tunnel: w1045 -> [_ _ _ w1182]
                  frame 0, Default {
                    n277 = for {
                      N: w1092 -> [_]
                      tunnel: w1089 -> [w1111]
                      tunnel: w1091 -> [w1109]
                      tunnel: [w1108] -> w1090
                      tunnel: [w1104] -> w1084 mode=indexing
                      tunnel: w1088 -> [w1106]
                      tunnel: w1087 -> [w1094]
                      tunnel: [w1096] -> w1086
                      tunnel: w1085 -> [w1095]
                      i -> [w1103]
                      stop <- w1108 stop-if-true
                      n278 = Index Array(array=w1111, index=w1103) -> (element=w1107:string)
                      n279 = Index Array(array=w1106, index=w1103) -> (element=w1105:string)
                      n280 = local write "STATUS"(w1105) -> ()
                      n281 = call "WSVCAP SHL Host TL RFFE Write - Multiple DUTs - Common Data.vi"("Data Out"=w1107, "error in"=w1094, "Log (T)"=FALSE) -> ("error out"=w1098:errorcluster)  [unwired: 12 in]
                      n282 = call "Delay T4.vi"("milliseconds to wait"=u32 10, "error in (no error)"=w1098) -> ("error out"=w1102:errorcluster)  [unwired: 9 in]
                      n283 = call "WS1050 AD7747 READ 36 DUT.vi"("error in"=w1102, "Log (T)"=w1095, "DUT Mask Mode (All)"=WSVCAP_SHL_I2C_DUT_Mask_Mode_Enum."C1") -> ("error out"=w1100:errorcluster, "AD7747 Values"=w1101:string[][])  [unwired: 7 in]
                      n284 = for {
                        tunnel: w1101 -> [w1114] mode=indexing
                        tunnel: w1100 -> [w1115]
                        tunnel: [w1115] -> w1096
                        tunnel: [w1112] -> w1104 mode=indexing
                        n285 = Index Array(array=w1114, index=1) -> (element=w1112:string)
                      }
                      n286 = Unbundle By Name(w1096) -> ("status"=w1110:bool)
                      n287 = Or(x=w1110, y=w1109) -> (x .or. y?=w1108:bool)
                    }
                  }
                  frame 1 {
                    n288 = for {
                      N: w1125 -> [_]
                      tunnel: w1122 -> [w1144]
                      tunnel: w1124 -> [w1142]
                      tunnel: [w1141] -> w1123
                      tunnel: [w1137] -> w1117 mode=indexing
                      tunnel: w1121 -> [w1139]
                      tunnel: w1120 -> [w1127]
                      tunnel: [w1129] -> w1119
                      tunnel: w1118 -> [w1128]
                      i -> [w1136]
                      stop <- w1141 stop-if-true
                      n289 = Index Array(array=w1144, index=w1136) -> (element=w1140:string)
                      n290 = Index Array(array=w1139, index=w1136) -> (element=w1138:string)
                      n291 = local write "STATUS"(w1138) -> ()
                      n292 = call "WSVCAP SHL Host TL RFFE Write - Multiple DUTs - Common Data.vi"("Data Out"=w1140, "error in"=w1127, "Log (T)"=FALSE) -> ("error out"=w1131:errorcluster)  [unwired: 12 in]
                      n293 = call "Delay T4.vi"("milliseconds to wait"=u32 10, "error in (no error)"=w1131) -> ("error out"=w1135:errorcluster)  [unwired: 9 in]
                      n294 = call "WS1050 AD7747 READ 36 DUT.vi"("error in"=w1135, "Log (T)"=w1128, "DUT Mask Mode (All)"=WSVCAP_SHL_I2C_DUT_Mask_Mode_Enum."C2") -> ("error out"=w1133:errorcluster, "AD7747 Values"=w1134:string[][])  [unwired: 7 in]
                      n295 = for {
                        tunnel: w1134 -> [w1147] mode=indexing
                        tunnel: w1133 -> [w1148]
                        tunnel: [w1148] -> w1129
                        tunnel: [w1145] -> w1137 mode=indexing
                        n296 = Index Array(array=w1147, index=3) -> (element=w1145:string)
                      }
                      n297 = Unbundle By Name(w1129) -> ("status"=w1143:bool)
                      n298 = Or(x=w1143, y=w1142) -> (x .or. y?=w1141:bool)
                    }
                  }
                  frame 2 {
                    n299 = for {
                      N: w1158 -> [_]
                      tunnel: w1155 -> [w1177]
                      tunnel: w1157 -> [w1175]
                      tunnel: [w1174] -> w1156
                      tunnel: [w1170] -> w1150 mode=indexing
                      tunnel: w1154 -> [w1172]
                      tunnel: w1153 -> [w1160]
                      tunnel: [w1162] -> w1152
                      tunnel: w1151 -> [w1161]
                      i -> [w1169]
                      stop <- w1174 stop-if-true
                      n300 = Index Array(array=w1177, index=w1169) -> (element=w1173:string)
                      n301 = Index Array(array=w1172, index=w1169) -> (element=w1171:string)
                      n302 = local write "STATUS"(w1171) -> ()
                      n303 = call "WSVCAP SHL Host TL RFFE Write - Multiple DUTs - Common Data.vi"("Data Out"=w1173, "error in"=w1160, "Log (T)"=FALSE) -> ("error out"=w1164:errorcluster)  [unwired: 12 in]
                      n304 = call "Delay T4.vi"("milliseconds to wait"=u32 10, "error in (no error)"=w1164) -> ("error out"=w1168:errorcluster)  [unwired: 9 in]
                      n305 = call "WS1050 AD7747 READ 36 DUT.vi"("error in"=w1168, "Log (T)"=w1161, "DUT Mask Mode (All)"=WSVCAP_SHL_I2C_DUT_Mask_Mode_Enum."C3") -> ("error out"=w1166:errorcluster, "AD7747 Values"=w1167:string[][])  [unwired: 7 in]
                      n306 = for {
                        tunnel: w1167 -> [w1180] mode=indexing
                        tunnel: w1166 -> [w1181]
                        tunnel: [w1181] -> w1162
                        tunnel: [w1178] -> w1170 mode=indexing
                        n307 = Index Array(array=w1180, index=1) -> (element=w1178:string)
                      }
                      n308 = Unbundle By Name(w1162) -> ("status"=w1176:bool)
                      n309 = Or(x=w1176, y=w1175) -> (x .or. y?=w1174:bool)
                    }
                  }
                  frame 3 {
                    n310 = for {
                      N: w1192 -> [_]
                      tunnel: w1183 -> [w1213]
                      tunnel: w1191 -> [w1211]
                      tunnel: [w1210] -> w1190
                      tunnel: [w1206] -> w1186 mode=indexing
                      tunnel: w1182 -> [w1208]
                      tunnel: w1187 -> [w1198]
                      tunnel: [w1194] -> w1185 mode=indexing
                      tunnel: [w1193] -> w1184 mode=indexing
                      shift-right: [w1199] -> w1188
                      shift-left: w1189 -> [w1197]
                      i -> [w1205]
                      stop <- w1210 stop-if-true
                      n311 = Index Array(array=w1213, index=w1205) -> (element=w1209:string)
                      n312 = Index Array(array=w1208, index=w1205) -> (element=w1207:string)
                      n313 = call "WSVCAP SHL Host TL RFFE Write - Multiple DUTs - Common Data.vi"("Data Out"=w1209, "error in"=w1197, "Log (T)"=FALSE) -> ("error out"=w1201:errorcluster)  [unwired: 12 in]
                      n314 = local write "STATUS"(w1207) -> ()
                      n315 = call "Delay T4.vi"("milliseconds to wait"=u32 10, "error in (no error)"=w1201) -> ("error out"=w1204:errorcluster)  [unwired: 9 in]
                      n316 = call "WS1050 AD7747 READ 36 DUT.vi"("error in"=w1204, "Log (T)"=w1198, "DUT Mask Mode (All)"=WSVCAP_SHL_I2C_DUT_Mask_Mode_Enum."All") -> ("error out"=w1203:errorcluster, "AD7747 Values"=w1195:string[][])  [unwired: 7 in]
                      n317 = for {
                        tunnel: w1195 -> [w1222] mode=indexing
                        tunnel: [w1220] -> w1206 mode=indexing
                        tunnel: w1195 -> [w1217] mode=indexing
                        tunnel: w1195 -> [w1216] mode=indexing
                        tunnel: [w1215] -> w1194 mode=indexing
                        tunnel: [w1214] -> w1193 mode=indexing
                        shift-right: [w1223] -> w1199
                        shift-left: w1203 -> [w1223]
                        n318 = Index Array(array=w1222, index=1) -> (element=w1220:string)
                        n319 = Index Array(array=w1217, index=3) -> (element=w1215:string)
                        n320 = Index Array(array=w1216, index=5) -> (element=w1214:string)
                      }
                      n321 = Unbundle By Name(w1199) -> ("status"=w1212:bool)
                      n322 = Or(x=w1212, y=w1211) -> (x .or. y?=w1210:bool)
                    }
                  }
                }
                n323 = Transpose 2D Array(2D array=w1053) -> (transposed array=w1063:string[][])
                "40V_1" <- w1063
                "NOM IDD ON (uA)" <- w1074
                "NOM IDD OFF(uA)" <- w1073
              }
              frame #2 {
                n324 = Array Size(array=w1245) -> (size(s)=w1246:i32)
                n325 = case shown="3" w1229 {
                  tunnel: w1246 -> [w1264 _ w1301]
                  tunnel: w1245 -> [w1263 _ w1300]
                  tunnel: w1244 -> [w1262 _ w1299]
                  tunnel: w1243 -> [w1261 w1290 w1298]
                  tunnel: [w1260 w1290 w1297] -> w1242
                  tunnel: [w1259 w1291 w1296] -> w1240
                  tunnel: w1238 -> [w1258 w1291 w1295]
                  tunnel: w1232 -> [w1257 _ w1294]
                  tunnel: [w1256 w1289 w1293] -> w1230
                  tunnel: w1226 -> [_ w1289 _]
                  tunnel: w1225 -> [w1255 w1288 w1292]
                  tunnel: [w1255 w1288 w1292] -> w1224
                  frame 0, 2, Default {
                    n326 = for {
                      N: w1264 -> [_]
                      tunnel: w1262 -> [w1283]
                      tunnel: w1261 -> [w1281]
                      tunnel: [w1280] -> w1260
                      tunnel: [w1276] -> w1256 mode=indexing
                      tunnel: w1263 -> [w1278]
                      tunnel: w1258 -> [w1266]
                      tunnel: [w1268] -> w1259
                      tunnel: w1257 -> [w1267]
                      i -> [w1275]
                      stop <- w1280 stop-if-true
                      n327 = Index Array(array=w1283, index=w1275) -> (element=w1279:string)
                      n328 = Index Array(array=w1278, index=w1275) -> (element=w1277:string)
                      n329 = call "WSVCAP SHL Host TL RFFE Write - Multiple DUTs - Common Data.vi"("Data Out"=w1279, "error in"=w1266, "Log (T)"=FALSE) -> ("error out"=w1270:errorcluster)  [unwired: 12 in]
                      n330 = local write "STATUS"(w1277) -> ()
                      n331 = call "Delay T4.vi"("milliseconds to wait"=u32 10, "error in (no error)"=w1270) -> ("error out"=w1274:errorcluster)  [unwired: 9 in]
                      n332 = call "WS1050 AD7747 READ 36 DUT.vi"("error in"=w1274, "Log (T)"=w1267, "DUT Mask Mode (All)"=WSVCAP_SHL_I2C_DUT_Mask_Mode_Enum."C2") -> ("error out"=w1272:errorcluster, "AD7747 Values"=w1273:string[][])  [unwired: 7 in]
                      n333 = for {
                        tunnel: w1273 -> [w1286] mode=indexing
                        tunnel: w1272 -> [w1287]
                        tunnel: [w1287] -> w1268
                        tunnel: [w1284] -> w1276 mode=indexing
                        n334 = Index Array(array=w1286, index=3) -> (element=w1284:string)
                      }
                      n335 = Unbundle By Name(w1268) -> ("status"=w1282:bool)
                      n336 = Or(x=w1282, y=w1281) -> (x .or. y?=w1280:bool)
                    }
                  }
                  frame 3 {
                  }
                  frame 1 {
                    n337 = for {
                      N: w1301 -> [_]
                      tunnel: w1299 -> [w1320]
                      tunnel: w1298 -> [w1318]
                      tunnel: [w1317] -> w1297
                      tunnel: [w1313] -> w1293 mode=indexing
                      tunnel: w1300 -> [w1315]
                      tunnel: w1294 -> [w1304]
                      shift-right: [w1305] -> w1296
                      shift-left: w1295 -> [w1303]
                      i -> [w1312]
                      stop <- w1317 stop-if-true
                      n338 = Index Array(array=w1320, index=w1312) -> (element=w1316:string)
                      n339 = Index Array(array=w1315, index=w1312) -> (element=w1314:string)
                      n340 = call "WSVCAP SHL Host TL RFFE Write - Multiple DUTs - Common Data.vi"("Data Out"=w1316, "error in"=w1303, "Log (T)"=FALSE) -> ("error out"=w1307:errorcluster)  [unwired: 12 in]
                      n341 = local write "STATUS"(w1314) -> ()
                      n342 = call "Delay T4.vi"("milliseconds to wait"=u32 10, "error in (no error)"=w1307) -> ("error out"=w1311:errorcluster)  [unwired: 9 in]
                      n343 = call "WS1050 AD7747 READ 36 DUT.vi"("error in"=w1311, "Log (T)"=w1304, "DUT Mask Mode (All)"=WSVCAP_SHL_I2C_DUT_Mask_Mode_Enum."C1") -> ("error out"=w1309:errorcluster, "AD7747 Values"=w1310:string[][])  [unwired: 7 in]
                      n344 = for {
                        tunnel: w1310 -> [w1323] mode=indexing
                        tunnel: [w1321] -> w1313 mode=indexing
                        shift-right: [w1324] -> w1305
                        shift-left: w1309 -> [w1324]
                        n345 = Index Array(array=w1323, index=1) -> (element=w1321:string)
                      }
                      n346 = Unbundle By Name(w1305) -> ("status"=w1319:bool)
                      n347 = Or(x=w1319, y=w1318) -> (x .or. y?=w1317:bool)
                    }
                  }
                }
                n348 = Transpose 2D Array(2D array=w1230) -> (transposed array=w1239:string[][])
                "40V_2" <- w1239
              }
              frame #3 {
                n349 = Array Size(array=w1344) -> (size(s)=w1345:i32)
                n350 = case shown="3" w1329 {
                  tunnel: w1345 -> [w1363 w1395 _]
                  tunnel: w1344 -> [w1362 w1394 _]
                  tunnel: w1343 -> [w1361 w1393 _]
                  tunnel: w1342 -> [w1360 w1392 w1421]
                  tunnel: [w1359 w1391 w1421] -> w1341
                  tunnel: w1336 -> [w1358 w1390 w1420]
                  tunnel: [w1357 w1389 w1420] -> w1328
                  tunnel: w1332 -> [w1356 w1388 _]
                  tunnel: [w1355 w1387 w1419] -> w1330
                  tunnel: w1325 -> [_ _ w1419]
                  frame 0, 1, Default {
                    n351 = for {
                      N: w1363 -> [_]
                      tunnel: w1361 -> [w1382]
                      tunnel: w1360 -> [w1380]
                      tunnel: [w1379] -> w1359
                      tunnel: [w1375] -> w1355 mode=indexing
                      tunnel: w1362 -> [w1377]
                      tunnel: w1356 -> [w1366]
                      shift-right: [w1367] -> w1357
                      shift-left: w1358 -> [w1365]
                      i -> [w1374]
                      stop <- w1379 stop-if-true
                      n352 = Index Array(array=w1382, index=w1374) -> (element=w1378:string)
                      n353 = Index Array(array=w1377, index=w1374) -> (element=w1376:string)
                      n354 = local write "STATUS"(w1376) -> ()
                      n355 = call "WSVCAP SHL Host TL RFFE Write - Multiple DUTs - Common Data.vi"("Data Out"=w1378, "error in"=w1365, "Log (T)"=FALSE) -> ("error out"=w1369:errorcluster)  [unwired: 12 in]
                      n356 = call "Delay T4.vi"("milliseconds to wait"=u32 10, "error in (no error)"=w1369) -> ("error out"=w1373:errorcluster)  [unwired: 9 in]
                      n357 = call "WS1050 AD7747 READ 36 DUT.vi"("error in"=w1373, "Log (T)"=w1366, "DUT Mask Mode (All)"=WSVCAP_SHL_I2C_DUT_Mask_Mode_Enum."C3") -> ("error out"=w1371:errorcluster, "AD7747 Values"=w1372:string[][])  [unwired: 7 in]
                      n358 = for {
                        tunnel: w1372 -> [w1385] mode=indexing
                        tunnel: [w1383] -> w1375 mode=indexing
                        shift-right: [w1386] -> w1367
                        shift-left: w1371 -> [w1386]
                        n359 = Index Array(array=w1385, index=5) -> (element=w1383:string)
                      }
                      n360 = Unbundle By Name(w1367) -> ("status"=w1381:bool)
                      n361 = Or(x=w1381, y=w1380) -> (x .or. y?=w1379:bool)
                    }
                  }
                  frame 2 {
                    n362 = for {
                      N: w1395 -> [_]
                      tunnel: w1393 -> [w1414]
                      tunnel: w1392 -> [w1412]
                      tunnel: [w1411] -> w1391
                      tunnel: [w1407] -> w1387 mode=indexing
                      tunnel: w1394 -> [w1409]
                      tunnel: w1390 -> [w1397]
                      tunnel: [w1399] -> w1389
                      tunnel: w1388 -> [w1398]
                      i -> [w1406]
                      stop <- w1411 stop-if-true
                      n363 = Index Array(array=w1414, index=w1406) -> (element=w1410:string)
                      n364 = Index Array(array=w1409, index=w1406) -> (element=w1408:string)
                      n365 = local write "STATUS"(w1408) -> ()
                      n366 = call "WSVCAP SHL Host TL RFFE Write - Multiple DUTs - Common Data.vi"("Data Out"=w1410, "error in"=w1397, "Log (T)"=FALSE) -> ("error out"=w1401:errorcluster)  [unwired: 12 in]
                      n367 = call "Delay T4.vi"("milliseconds to wait"=u32 10, "error in (no error)"=w1401) -> ("error out"=w1405:errorcluster)  [unwired: 9 in]
                      n368 = call "WS1050 AD7747 READ 36 DUT.vi"("error in"=w1405, "Log (T)"=w1398, "DUT Mask Mode (All)"=WSVCAP_SHL_I2C_DUT_Mask_Mode_Enum."C1") -> ("error out"=w1403:errorcluster, "AD7747 Values"=w1404:string[][])  [unwired: 7 in]
                      n369 = for {
                        tunnel: w1404 -> [w1417] mode=indexing
                        tunnel: w1403 -> [w1418]
                        tunnel: [w1418] -> w1399
                        tunnel: [w1415] -> w1407 mode=indexing
                        n370 = Index Array(array=w1417, index=1) -> (element=w1415:string)
                      }
                      n371 = Unbundle By Name(w1399) -> ("status"=w1413:bool)
                      n372 = Or(x=w1413, y=w1412) -> (x .or. y?=w1411:bool)
                    }
                  }
                  frame 3 {
                  }
                }
                n373 = Transpose 2D Array(2D array=w1330) -> (transposed array=w1337:string[][])
                "40V_3" <- w1337
              }
              frame #4 {
                # "VPI Testing @ 35V"
                n374 = call "WS1050 Delta C Calculation.vi"("error in (no error)"=w1461, "DCap Target(pF)"=w1460, "Input"=w1463) -> ("error out"=w1458:errorcluster, "Total Bank Delta C(pF)"=w1451:string[], "% Bank DeltaC"=w1455:string[])  [unwired: 4 in, 2 out]
                n375 = call "WS1050 Delta C Calculation.vi"("error in (no error)"=w1461, "DCap Target(pF)"=w1460, "Input"=w1462) -> ("error out"=w1459:errorcluster, "Total Bank Delta C(pF)"=w1450:string[], "% Bank DeltaC"=w1453:string[])  [unwired: 4 in, 2 out]
                n376 = call "WS1050 Delta C Calculation.vi"("error in (no error)"=w1461, "DCap Target(pF)"=w1460, "Input"=w1454) -> ("error out"=w1457:errorcluster, "Total Bank Delta C(pF)"=w1449:string[], "% Bank DeltaC"=w1452:string[])  [unwired: 4 in, 2 out]
                n377 = Merge Errors(w1458, w1459, w1457) -> (w1456:errorcluster)
                n378 = case shown="1, Default" w1464 {
                  tunnel: w1456 -> [w1491 w1499]
                  tunnel: [w1491 w1499] -> w1429
                  tunnel: w1455 -> [w1487 w1495]
                  tunnel: w1453 -> [w1486 w1494]
                  tunnel: w1452 -> [w1485 w1493]
                  tunnel: w1451 -> [w1490 w1498]
                  tunnel: [w1490 w1498] -> w1448
                  tunnel: w1450 -> [w1489 w1497]
                  tunnel: [w1489 w1497] -> w1447
                  tunnel: w1449 -> [w1488 w1496]
                  tunnel: [w1488 w1496] -> w1446
                  frame 0 {
                    n379 = Build Array(w1487, w1486, w1485) -> (→"% Delta C_T0":string[][])
                  }
                  frame 1, Default {
                    n380 = Build Array(w1495, w1494, w1493) -> (→"% Delta C":string[][])
                  }
                }
                "Total Delta C1(pF)" <- w1448
                "Total Delta C2(pF)" <- w1447
                "Total Delta C3(pF)" <- w1446
                n381 = call "WS1050_51 VPI Header_Ver1.4.vi"("VPI Name"="VPI Name", "VPI_Cmd"="VPI_Cmd", "Cmin/Act"=w1427, "WS1050/51"=w1432, "error in (no error)"=w1433) -> ("VPI Header"=w1431:string[], "VPI_ALL"=w1426:string[], "Cmd_ALL"=w1425:string[], "error out"=w1430:errorcluster)  [unwired: 7 in]
                n382 = Merge Errors(w1430, w1429) -> (w1428:errorcluster)
                n383 = case shown="True" w1438 {
                  tunnel: w1475 -> [w1506 w1514]
                  tunnel: [w1502 w1516] -> w1442
                  tunnel: [w1500 w1513] -> w1424
                  tunnel: [w1500 w1531] -> w1422
                  tunnel: [w1506 w1514] -> w1473
                  tunnel: w1470 -> [w1508 w1535]
                  tunnel: [w1508 w1535] -> w1469
                  tunnel: w1425 -> [_ w1534]
                  tunnel: [w1500 w1515] -> w1423
                  tunnel: w1426 -> [w1505 w1532]
                  tunnel: ["NA" ("string") w1530] -> w1444
                  tunnel: w1428 -> [w1503 w1525]
                  frame False {
                    n384 = Array Size(array=w1505) -> (size(s)=w1504:i32)
                    n385 = for {
                      N: w1504 -> [_]
                      tunnel: [w1510] -> w1501 mode=indexing
                      shift-right: [w1509] -> w1502
                      shift-left: w1503 -> [w1509]
                      n386 = for {
                        N: 36 -> [_]
                        tunnel: ["na"] -> w1510 mode=indexing
                      }
                    }
                    n387 = Transpose 2D Array(2D array=w1501) -> (transposed array=w1500:string[][])
                  }
                  frame True {
                    w1527 = FALSE ("Log (T)")
                    # "Set CP to 35V"
                    n388 = call "WSVCAP SHL Host TL RFFE Write - Multiple DUTs - Common Data.vi"("Data Out"="074820", "error in"=w1525, "Log (T)"=w1527) -> ("error out"=w1523:errorcluster)  [unwired: 12 in]
                    n389 = call "Delay T4.vi"("milliseconds to wait"=u32 10, "error in (no error)"=w1523) -> ("error out"=w1528:errorcluster)  [unwired: 9 in]
                    n390 = case shown="3" "CP VPI" {
                      selector: "CP VPI" -> [w1540 w1545 w1550 w1554]
                      tunnel: string[] ["07476F", "074776", "074765", "074769", "07477B"] -> [w1541 w1546 w1551 w1556]
                      tunnel: [w1539 w1544 w1549 w1555] -> w1521
                      tunnel: [w1537 w1542 w1547 w1552] -> w1520
                      tunnel: ["35" ("string") "27.5" ("string") "30.5" ("string") "40.25" ("string")] -> w1530
                      tunnel: w1528 -> [w1537 w1542 w1547 w1552]
                      frame 0, Default {
                        n391 = Index Array(array=w1541, index=w1540) -> (element=w1539:string)
                      }
                      frame 2 {
                        n392 = Index Array(array=w1546, index=w1545) -> (element=w1544:string)
                      }
                      frame 3 {
                        n393 = Index Array(array=w1551, index=w1550) -> (element=w1549:string)
                      }
                      frame 1 {
                        n394 = Index Array(array=w1556, index=w1554) -> (element=w1555:string)
                      }
                    }
                    n395 = Array Size(array=w1532) -> (size(s)=w1536:i32)
                    n396 = call "WSVCAP SHL Host TL RFFE Write - Multiple DUTs - Common Data.vi"("Data Out"=w1521, "error in"=w1520, "Log (T)"=w1527) -> ("error out"=w1529:errorcluster)  [unwired: 12 in]
                    n397 = for {
                      N: w1536 -> [_]
                      tunnel: w1534 -> [w1577]
                      tunnel: w1514 -> [w1575]
                      tunnel: [w1572] -> w1533 mode=indexing
                      tunnel: w1532 -> [w1571]
                      tunnel: w1529 -> [w1561]
                      tunnel: [w1563] -> w1516
                      tunnel: [w1559] -> w1518 mode=indexing
                      tunnel: [w1557] -> w1517 mode=indexing
                      i -> [w1570]
                      stop <- w1574 stop-if-true
                      n398 = Index Array(array=w1577, index=w1570) -> (element=w1573:string)
                      n399 = Index Array(array=w1571, index=w1570) -> (element=w1569:string)
                      n400 = local write "STATUS"(w1569) -> ()
                      n401 = call "WSVCAP SHL Host TL RFFE Write - Multiple DUTs - Common Data.vi"("Data Out"=w1573, "error in"=w1561, "Log (T)"=FALSE) -> ("error out"=w1568:errorcluster)  [unwired: 12 in]
                      n402 = call "Delay T4.vi"("milliseconds to wait"=u32 10, "error in (no error)"=w1568) -> ("error out"=w1565:errorcluster)  [unwired: 9 in]
                      n403 = call "WS1050 AD7747 READ 36 DUT.vi"("error in"=w1565, "Log (T)"=FALSE, "DUT Mask Mode (All)"=WSVCAP_SHL_I2C_DUT_Mask_Mode_Enum."All") -> ("error out"=w1566:errorcluster, "AD7747 Values"=w1558:string[][])  [unwired: 7 in]
                      n404 = for {
                        tunnel: [w1586] -> w1572 mode=indexing
                        tunnel: w1566 -> [w1585]
                        tunnel: [w1585] -> w1563
                        tunnel: w1558 -> [w1584] mode=indexing
                        tunnel: w1558 -> [w1582] mode=indexing
                        tunnel: [w1581] -> w1559 mode=indexing
                        tunnel: w1558 -> [w1579] mode=indexing
                        tunnel: [w1578] -> w1557 mode=indexing
                        n405 = Index Array(array=w1579, index=5) -> (element=w1578:string)
                        n406 = Index Array(array=w1584, index=1) -> (element=w1586:string)
                        n407 = Index Array(array=w1582, index=3) -> (element=w1581:string)
                      }
                      n408 = Unbundle By Name(w1563) -> ("status"=w1576:bool)
                      n409 = Or(x=w1576, y=w1575) -> (x .or. y?=w1574:bool)
                    }
                    n410 = Transpose 2D Array(2D array=w1533) -> (transposed array=w1513:string[][])
                    n411 = Transpose 2D Array(2D array=w1518) -> (transposed array=w1515:string[][])
                    n412 = Transpose 2D Array(2D array=w1517) -> (transposed array=w1531:string[][])
                  }
                }
                "VPI C1" <- w1424
                "VPI C3" <- w1422
                "VPI C2" <- w1423
                n413 = Insert Into Array(array=w1466, new element=w1431) -> (w1465:string[])  [unwired: 1 in]
                n414 = case shown="True" w1443 {
                  tunnel: w1442 -> [w1477 w1482]
                  tunnel: [w1478 w1481] -> w1441
                  frame False {
                    n415 = call "WSVCAP SHL Host TL RFFE Write - Multiple DUTs - Common Data.vi"("Data Out"="074820", "error in"=w1477, "Log (T)"=FALSE) -> ("error out"=w1478:errorcluster)  [unwired: 12 in]
                  }
                  frame True {
                    n416 = call "WSVCAP SHL Host TL RFFE Write - Multiple DUTs - Common Data.vi"("Data Out"="074800", "error in"=w1482, "Log (T)"=FALSE) -> ("error out"=w1481:errorcluster)  [unwired: 12 in]
                  }
                }
                n417 = call "Delay T4.vi"("milliseconds to wait"=u32 10, "error in (no error)"=w1441) -> ("error out"=w1440:errorcluster)  [unwired: 9 in]
              }
              frame #5 {
                # "VSA Testing"
                n418 = case shown="True" w1588 {
                  tunnel: w1627 -> [w1639 w1653]
                  tunnel: [w1638 w1652] -> w1601
                  tunnel: [w1643 w1659] -> w1617
                  tunnel: w1618 -> [w1643 w1658]
                  tunnel: [w1640 w1656] -> w1606
                  tunnel: [w1640 w1655] -> w1603
                  tunnel: [w1640 w1654] -> w1600
                  tunnel: [w1641 w1657] -> w1607
                  frame False {
                    n419 = for {
                      tunnel: dbl[] [0.0, 0.0, 0.0] -> [w1648] mode=indexing
                      tunnel: [w1647] -> w1641 mode=indexing
                      tunnel: [w1645] -> w1640 mode=indexing
                      shift-right: [w1644] -> w1638
                      shift-left: w1639 -> [w1644]
                      w1646 = 36
                      n420 = Number To Fractional String(number=w1648) -> (F-format string=w1649:string)  [unwired: 3 in]
                      n421 = for {
                        N: w1646 -> [_]
                        tunnel: w1649 -> [w1651]
                        tunnel: [w1651] -> w1647 mode=indexing
                      }
                      n422 = for {
                        N: w1646 -> [_]
                        tunnel: ["na"] -> w1645 mode=indexing
                      }
                    }
                  }
                  frame True {
                    n423 = for {
                      tunnel: "VSA Voltage(V)" -> [w1677] mode=indexing
                      tunnel: [w1681] -> w1659
                      tunnel: w1658 -> [w1679]
                      tunnel: [w1678] -> w1656 mode=indexing
                      tunnel: [w1666] -> w1655 mode=indexing
                      tunnel: [w1674] -> w1657 mode=indexing
                      tunnel: [w1665] -> w1654 mode=indexing
                      shift-right: [w1664] -> w1652
                      shift-left: w1653 -> [w1668]
                      w1673 = u16 0 items=["Voltage", "Current"] ("Source Mode  (0: Voltage)")
                      n424 = call "Configure Output.vi"("Source Mode  (0: Voltage)"=w1673, "error in (no error)"=w1668, "Compliance  Level (0.1)"=0.1, "Output Level (0)"=w1677, "VISA resource name"=w1679) -> ("error out"=w1685:errorcluster, "VISA resource name out"=w1683:refnum<visa-resource-name>)  [unwired: 5 in]
                      n425 = Number To Fractional String(number=w1677) -> (F-format string=w1676:string)  [unwired: 3 in]
                      n426 = call "Enable Output.vi"("error in (no error)"=w1685, "Enable Output (T: Enable)"=TRUE, "VISA resource name"=w1683) -> ("error out"=w1686:errorcluster, "VISA resource name out"=w1681:refnum<visa-resource-name>)  [unwired: 7 in]
                      n427 = call "Delay T4.vi"("milliseconds to wait"=u32 50, "error in (no error)"=w1686) -> ("error out"=w1672:errorcluster)  [unwired: 9 in]
                      n428 = for {
                        N: 36 -> [_]
                        tunnel: w1676 -> [w1687]
                        tunnel: [w1687] -> w1674 mode=indexing
                      }
                      n429 = call "WS1050 AD7747 READ 36 DUT.vi"("error in"=w1672, "Log (T)"=FALSE, "DUT Mask Mode (All)"=WSVCAP_SHL_I2C_DUT_Mask_Mode_Enum."All") -> ("error out"=w1669:errorcluster, "AD7747 Values"=w1671:string[][])  [unwired: 7 in]
                      n430 = for {
                        tunnel: w1671 -> [w1690] mode=indexing
                        tunnel: [w1694] -> w1678 mode=indexing
                        shift-right: [w1693] -> w1663
                        shift-left: w1669 -> [w1693]
                        tunnel: [w1689] -> w1666 mode=indexing
                        tunnel: [w1688] -> w1665 mode=indexing
                        n431 = Index Array(array=w1690, index=3) -> (element=w1689:string)
                        n432 = Index Array(array=w1690, index=5) -> (element=w1688:string)
                        n433 = Index Array(array=w1690, index=1) -> (element=w1694:string)
                      }
                      n434 = call "Delay T4.vi"("milliseconds to wait"=u32 50, "error in (no error)"=w1663) -> ("error out"=w1664:errorcluster)  [unwired: 9 in]
                    }
                    n435 = local write "STATUS"("VSA Testing...." ("STATUS")) -> ()
                  }
                }
                n436 = Transpose 2D Array(2D array=w1607) -> (transposed array=w1605:string[][])
                n437 = Transpose 2D Array(2D array=w1606) -> (transposed array=w1604:string[][])
                n438 = Transpose 2D Array(2D array=w1603) -> (transposed array=w1602:string[][])
                n439 = Transpose 2D Array(2D array=w1600) -> (transposed array=w1599:string[][])
                n440 = call "WS1050_VSA_Convert_Data.vi"("VSA_C3"=w1599, "error in (no error)"=w1601, "VSA_C2"=w1602, "VSA_C1"=w1604, "Voltage"=w1605) -> ("error out"=w1598:errorcluster, "VSA_V3"=w1595:string[][], "VSA_V2"=w1596:string[][], "VSA_V1"=w1597:string[][])  [unwired: 3 in]
                "VSA_V1" <- w1597
                "VSA_V2" <- w1596
                "VSA_V3" <- w1595
                n441 = case shown="True" w1588 {
                  tunnel: w1617 -> [w1631 w1637]
                  tunnel: [w1631 w1636] -> w1616
                  tunnel: w1598 -> [w1630 w1635]
                  tunnel: [w1630 w1632] -> w1615
                  frame False {
                  }
                  frame True {
                    w1633 = u16 0 items=["Voltage", "Current"] ("Source Mode  (0: Voltage)")
                    n442 = call "Configure Output.vi"("Source Mode  (0: Voltage)"=w1633, "error in (no error)"=w1635, "Output Level (0)"=0.0, "VISA resource name"=w1637) -> ("error out"=w1632:errorcluster, "VISA resource name out"=w1636:refnum<visa-resource-name>)  [unwired: 6 in]
                  }
                }
                n443 = call "Delay T4.vi"("milliseconds to wait"=u32 50, "error in (no error)"=w1615) -> ("error out"=w1614:errorcluster)  [unwired: 9 in]
              }
              frame #6 {
                # "Handshake Check and EFuse Readback"
                n444 = Or(x=w1704, y=w1714) -> (x .or. y?=w1713:bool)
                n445 = Add(x=w1726, y=w1725) -> (x+y=w1712:u64)
                n446 = case shown="False" w1713 {
                  tunnel: w1739 -> [w1752 _]
                  tunnel: w1738 -> [w1751 w1757]
                  tunnel: [w1750 w1757] -> w1737
                  tunnel: w1736 -> [w1749 _]
                  tunnel: w1735 -> [w1748 _]
                  tunnel: w1734 -> [w1747 _]
                  tunnel: [w1743 w1756] -> w1733
                  tunnel: [w1742 w1756] -> w1728
                  tunnel: w1712 -> [w1741 _]
                  tunnel: w1719 -> [w1740 _]
                  frame False {
                    n447 = call "WS1050_36DUT_Handshake Check R1_Record All Regs Ver1.0.vi"("file path (use dialog)"=w1752, "Reg1_Bit Cntrl"="Reg1_Bit Cntrl", "File Name"=w1740, "SN"=w1747, "Loop"=w1741, "error"=w1751, "Lot #"=w1749, "Wafer #"=w1748) -> ("Pass/Fail"=→"EFuse Readback Status":bool[], "EFuse Read back"=w1742:string[], "Status"=w1743:string[], "error out"=w1750:errorcluster)  [unwired: 6 in, 2 out]
                    n448 = case shown="1, Default" w1741 {
                      tunnel: w1742 -> [w1753 w1754]
                      frame 0 {
                        "EFuse RB T0" <- w1753
                      }
                      frame 1, Default {
                        "Current EFuse Read back" <- w1754
                      }
                    }
                    n449 = local write "STATUS"("Hand Shake & EFuse Readback...." ("STATUS")) -> ()
                  }
                  frame True {
                    n450 = for {
                      N: 36 -> [_]
                      tunnel: ["na"] -> w1756 mode=indexing
                    }
                  }
                }
                n451 = Add(x=w1712, y=w1709) -> (x+y=w1710:u64)
                "TTCompleted" <- w1710
                n452 = Number To Engineering String(4:w1710) -> (0:w1724:string)  [unwired: 3 in]
                n453 = Build Array(w1723, w1721, w1720) -> (w1722:string[])
              }
              frame #7 {
                # "Save Data"
                n454 = Increment(x=w1769) -> (x+1=w1768:i32)
                n455 = local write "STATUS"("Saving Data...." ("STATUS")) -> ()
                n456 = Multiply(x=w1768, y=36) -> (x*y=w1763:i32)
                n457 = Path To String(path=w1773) -> (string=w1772:string)
                n458 = Bundle("Test Program"=w1805, "Comment"=w1804, "Data Out"=w1780, "Data Out"=w1779, "Data Out"=w1778, w1777, "Data Out"=w1776, "Data Out"=w1775, "string"=w1774, "Freq(Hz)"=w1761, "Board#"=w1759) -> (w1760:T8)  [unwired: 1 in]
                n459 = case shown="True" "Debug" {
                  tunnel: w1763 -> [w1812 w1815]
                  tunnel: [w1812 w1813] -> w1762
                  frame False {
                  }
                  frame True {
                    n460 = Multiply(x=w1815, y="No of Rows\nFrom Spread Sheet") -> (x*y=w1813:i32)
                  }
                }
                n461 = call "WS1050_36 DUT SData Ver1.0.vi"("TMN DC\\CAP Data Log File Path"=w1773, "Lot#"=w1807, "Total Delta C1(pF)"=w1783, "VSA_V1"=w1792, "Wafer#"=w1803, "File Name"=w1766, "Total Delta C2(pF)"=w1782, "error in"=w1810, "TP/Comment"=w1760, "EFuse"=w1797, "Data Output C3"=w1785, "Temperature"=w1789, "VSA_V2"=w1793, "VPI C3"=w1787, "Data Output C1"=w1800, "VPI C2"=w1786, "SN"=w1808, "R/W Status"=w1806, "Cap Header"=w1788, "HD/Cycles Completed"=w1796, "Data Output C2"=w1784, "VSA_V3"=w1791, "Current"=w1799, "VPI C1"=w1798, "Total Delta C3(pF)"=w1781) -> ("error out"=w1809:errorcluster)  [unwired: 2 in]
                n462 = Concatenate Strings(w1772, "\\" ("string"), w1766, "_Multi Socket Data.csv" ("string")) -> (w1771:string)
              }
              frame #8 {
                n463 = case shown="True" "Plot Delta Cmin" {
                  tunnel: w1820 -> [w1835 w1850]
                  tunnel: [w1835 w1846] -> w1819
                  tunnel: w1818 -> [_ w1842]
                  tunnel: w1816 -> [_ w1840]
                  frame False {
                  }
                  frame True {
                    w1836 = 2 items=["C1", "C2", "C3", "D_C1", "D_C2", "D_C3"] ("Bank")
                    w1837 = 1 items=["C1", "C2", "C3", "D_C1", "D_C2", "D_C3"] ("Bank")
                    w1838 = 0 items=["C1", "C2", "C3", "D_C1", "D_C2", "D_C3"] ("Bank")
                    n464 = String To Path(string=w1842) -> (path=w1841:path)
                    n465 = call "Delay T4.vi"("milliseconds to wait"=u32 50, "error in (no error)"=w1850) -> ("error out"=w1849:errorcluster)  [unwired: 9 in]
                    n466 = call "36DUT Plot From Spread Sheet.vi"("Plot"="Plot", "No of Rows"=w1840, "error in (no error)"=w1849, "Bank"=w1838, "file path (dialog if empty)"=w1841) -> ("error out"=w1844:errorcluster, "Delta C_Min Plot"=→"Min Plot_1":dbl[][])  [unwired: 5 in]
                    n467 = call "36DUT Plot From Spread Sheet.vi"("Plot"="Plot", "No of Rows"=w1840, "error in (no error)"=w1844, "Bank"=w1837, "file path (dialog if empty)"=w1841) -> ("error out"=w1845:errorcluster, "Delta C_Min Plot"=→"Min Plot_2":dbl[][])  [unwired: 5 in]
                    n468 = call "36DUT Plot From Spread Sheet.vi"("Plot"="Plot", "No of Rows"=w1840, "error in (no error)"=w1845, "Bank"=w1836, "file path (dialog if empty)"=w1841) -> ("error out"=w1846:errorcluster, "Delta C_Min Plot"=→"Min Plot_3":dbl[][])  [unwired: 5 in]
                  }
                }
                n469 = Get Date/Time In Seconds() -> (seconds since 1Jan1904=w1828:timestamp)
                n470 = Get Date/Time String(seconds (now)=w1828, want seconds? (F)=TRUE) -> (date string=→"date string":string, time string=→"Previous Time":string)  [unwired: 1 in]
                n471 = Greater Or Equal?(x=w1825, y="Set HD/Cycle \nto Complete") -> (x >= y?=w1832:bool)
                n472 = Greater Or Equal?(x=w1824, y="TTF Completed") -> (x >= y?=w1823:bool)
                "No of HD/Cycle\nCompleted" <- w1825
              }
            }
            n473 = Increment(x=w582) -> (x+1=→"Loop \ncompleted":i32)
            n474 = call "Delay T4.vi"("milliseconds to wait"=u32 10, "error in (no error)"=w469) -> ("error out"=w470:errorcluster)  [unwired: 9 in]
            n475 = Compound Arithmetic op=OR(w651, w552, w578) -> (w591:bool)
          }
          "Total Time" <- w409
          n476 = Increment(x=w407) -> (x+1=→"Run Loops":i32)
          n477 = local write "No of HD/Cycle\nCompleted"(u64 0 ("No of HD/Cycle\nCompleted")) -> ()
          n478 = Unbundle By Name(w399) -> ("status"=w413:bool)
          n479 = Compound Arithmetic op=OR(w413, w405, w404) -> (w395:bool)
        }
        n480 = for {
          tunnel: w291 -> [w1862]
          tunnel: w269 -> [w1861]
          tunnel: w320 -> [w1859] mode=indexing
          tunnel: [w1854] -> w289
          tunnel: [w1858] -> w319
          n481 = call "E3631A_Voltage Controller.vi"("VISA resource name"=w1861, "I_VDD(A)"=0.5, "Channel Controller"=w1859, "Voltage 1"=0.0, "Voltage 2"=3.3, "error in (no error)"=w1862, "I_3.3V (A)"=0.5) -> ("VISA resource name out"=w1858:refnum<visa-resource-name>, "error out"=w1855:errorcluster)  [unwired: 7 in]
          n482 = call "Delay T4.vi"("milliseconds to wait"=u32 100, "error in (no error)"=w1855) -> ("error out"=w1854:errorcluster)  [unwired: 9 in]
        }
        n483 = VISA Write(VISA resource name=w310, write buffer="SOUR:FUNC VOLT;VOLT:MODE FIX;RANG 100;LEV 0.0;:SENS:FUNC \"CURR\";CURR:PROT 60E-3;RANG 100E-3;:OUTP ON", error in (no error)=w291) -> (VISA resource name out=w308:refnum<visa-resource-name>, error out=w290:errorcluster)  [unwired: 1 out]
        n484 = Merge Errors(w289, w290) -> (w309:errorcluster)
      }
      frame True {
      }
    }
    n485 = local write "stop During HD/Cycles"(w70) -> ()
    n486 = Wait Until Next ms Multiple(millisecond multiple=u32 100) -> ()  [unwired: 1 out]
    n487 = Unbundle By Name(w71) -> ("status"=w89:bool)
    n488 = Or(x=w89, y=w80) -> (x .or. y?=w88:bool)
    "STATUS" <- "Idle...." ("STATUS")
  }
  "Ke2000 Out" <- w22
  "PS1 Out" <- w21
  n489 = local write "stop During HD/Cycles"(w7) -> ()
  n490 = local write "stop"(w7) -> ()
  n491 = VISA Write(VISA resource name=w14, write buffer="SOUR:FUNC VOLT;VOLT:MODE FIX;RANG 100;LEV 0.0;:SENS:FUNC \"CURR\";CURR:PROT 60E-3;RANG 100E-3;:OUTP OFF", error in (no error)=w13) -> (VISA resource name out=→"VISA resource name out":refnum<visa-resource-name>, error out=→"error out 2":errorcluster)  [unwired: 1 out]
  n492 = case shown="True" w19 {
    tunnel: [w1879 w1882] -> w2
    tunnel: w13 -> [w1879 w1881]
    frame False {
    }
    frame True {
      n493 = local write "Online"(FALSE ("Online")) -> ()
      n494 = call "WSVCAP SHL Host TL Close.vi"("error in"=w1881) -> ("error out"=w1882:errorcluster)  [unwired: 14 in]
    }
  }
  "error out" <- w2
